vi "XY_plot_gnuplot.vi"(0 "Plot Array":cluster{dbl[], dbl[]}[](array[cluster])=[{[500.0, 500.0, 953.54, 215.0, 270.0, 320.0, 445.0, 525.0, 600.0, 675.0, 750.0, 825.0, 900.0, 960.0, 1010.0, 1060.0], [4.614524, 4.54365, 5.818368, 0.1374656, 0.6662545, 1.465458, 3.619824, 4.848976, 5.887329, 5.940571, 6.152151, 5.717487, 5.600293, 5.40069, 5.154843, 5.121789]}, {[100.0, 150.0, 215.0, 270.0, 320.0, 445.0, 525.0, 600.0, 675.0, 750.0, 825.0, 900.0, 960.0, 1010.0, 1060.0], [0.002314715, -0.00693192, 0.120417, 0.6880509, 1.519176, 3.513709, 5.065183, 6.116033, 6.096773, 5.938465, 5.593788, 5.5597, 5.387002, 5.304077, 4.887903]}] {"?" format="%.2f"; "?" format="%.2f"}, 1 "Job Directory":path=path "/G4_2_HD/Users/paulhayden/Documents/Projects/Westlakes_resolution") -> (2 "Saved Automatically?":bool, 3 "Tex Info String":string="set term epslatex\nset output \"Plot.eps\"\nset xlabel '$Distance~(m)$'\nset ylabel '$DF~(s/m^3)\\times10^6$'\nset samples 1000\nset pointsize 1.00\nset title '$B38~Centreline~Glc$' 0, 0\nset size 0.75,0.9\n\n#set key 450, -2.5833\n unset key\nset label 1 '~~~~~~~~~~~Angle~(deg)~=~0' at -100, -2.58\nset label 2 '~~~~~~~~~~~Height~(m)~=~5' at -100, -3.27\n set xrange [0 : 500] \n# set autoscale x \n set yrange [0.10000 : 7]\n# set autoscale y \n\nplot \"B38_Centreline_Glc.dat\" index 0 using 1:2 axes x1y1 title '$File=B38R~DDD.xls$' with points 1 1, \\\n\"B38_Centreline_Glc.dat\" index 1 using 1:2 axes x1y1 title '$File=B38R~DDD~1.xls$' with points 1 3", 4 "Plot data file":path)   [LabVIEW 2011]
uses:
  Gnuplot_Label.ctl
  Results_plotter_Global.vi
  <vilib>/Analysis/NI_AALBase.lvlib
  <vilib>/Analysis/NI_AALPro.lvlib
panel:
  in  "Fixed Zp":dbl format="%.2f"
  in  "Auto Zp":bool=TRUE
  in  "Put Coeff\nin Results file":bool
  in  "Case Constant\n(See Context Help)":bool
  in  "Minor Gridlines":T1(ring)
  in  "Major Gridlines":T1(ring)
  in  "Legend Position":u16(ring) items=["Auto", "top left", "top right", "bottom left", "bottom right"]
  in  "Ymax":bool=TRUE
  in  "Ymax Val":dbl
  in  "Xmax":bool=TRUE
  in  "Xmax Val":dbl
  in  "Xmin":bool=TRUE
  in  "Xmin Val":dbl
  in  "Ymin":bool=TRUE
  in  "X Log?":bool
  out "Time format?":bool
  in  "plot error bars?":bool
  out "Path":path
  in  "Show Labels?":bool
  in  "Ymin Val":dbl
  out "Final Title":string="B38 Centreline Glc"
  in  "y Log?":bool
  in  "Show Re-Run Gnuplot?":bool
  in  "Mode":T2
  in  "Wavelength?":bool
  in  "Separation":dbl=1.2
  in  "Reverse order":bool
  in  "Offset?":bool
  out "Extra range":dbl
  in  "precision":string
  out "Profile offset":dbl
  in  "Graph Height":string="0.9"
  in  "Graph width":string="0.75"
  in  "Filename Max length":i32=28
  in  "Save data analysis file":bool
  in  "Plot Title":u16(ring) items=["Title String Only", "Number of Measurements", "Date:of:Measurement", "Time:Measurement:Commenced", "Seconds:since:1st Jan", "Time::", "Raw:Data:Filename", "w1Demeaned::", "w2Demeaned::", "w3Demeaned::", "w5Demeaned::", "Ch 1:Mean:Gen (w1)", "Ch 1:Variance:Gen (w1)", "Ch 2:Mean:Gen (w2)", "Ch 2:Variance:Gen (w2)", "Ch 3:Mean:Gen (w3)", "Ch 3:Variance:Gen (w3)", "Ch 4:Mean:Gen (w5)", "Ch 4:Variance:Gen (w5)", "Tunnel3:SettlingChamber:Temperature(C)"]
  in  "Plot style":u16[](array[ring])=[0, 0, 0, 0, 0, 0, 0, 0, 0, 0, 0] items=["points", "lines", "linespoints"]
  in  "Summarise":u16(ring) items=["All Series", "w1Demeaned__", "w2Demeaned__", "w3Demeaned__", "w5Demeaned__"]
  in  "Added labels":i32[](listbox)
  out "Delta y":dbl=0.6900000000000001
  out "Y location":dbl=-2.583333333333333
  out "X location":dbl=-100.0
  in  "Plot Title":string
  in  "Show legend?":bool
  in  "Point Size":dbl=1.2 format="%.2f"
  out "No of Series":i32=2
  in  "Fit type":T3(ring)
  out "No Legend":i32=397
  out "With legend":i32=580
  in  "Save Automatically?":bool
  in  "Analysis":T4(ring)
  out "XY Graph":cluster{dbl[], dbl[]}[](graph)=[{[215.0, 270.0, 320.0, 445.0, 500.0, 500.0, 525.0, 600.0, 675.0, 750.0, 825.0, 900.0, 953.54, 960.0, 1010.0, 1060.0], [0.1374656, 0.6662545, 1.465458, 3.619824, 4.614524, 4.54365, 4.848976, 5.887329, 5.940571, 6.152151, 5.717487, 5.600293, 5.818368, 5.40069, 5.154843, 5.121789]}, {[100.0, 150.0, 215.0, 270.0, 320.0, 445.0, 525.0, 600.0, 675.0, 750.0, 825.0, 900.0, 960.0, 1010.0, 1060.0], [0.002314715, -0.00693192, 0.120417, 0.6880509, 1.519176, 3.513709, 5.065183, 6.116033, 6.096773, 5.938465, 5.593788, 5.5597, 5.387002, 5.304077, 4.887903]}]
  # "Scales"
  # "Auto"
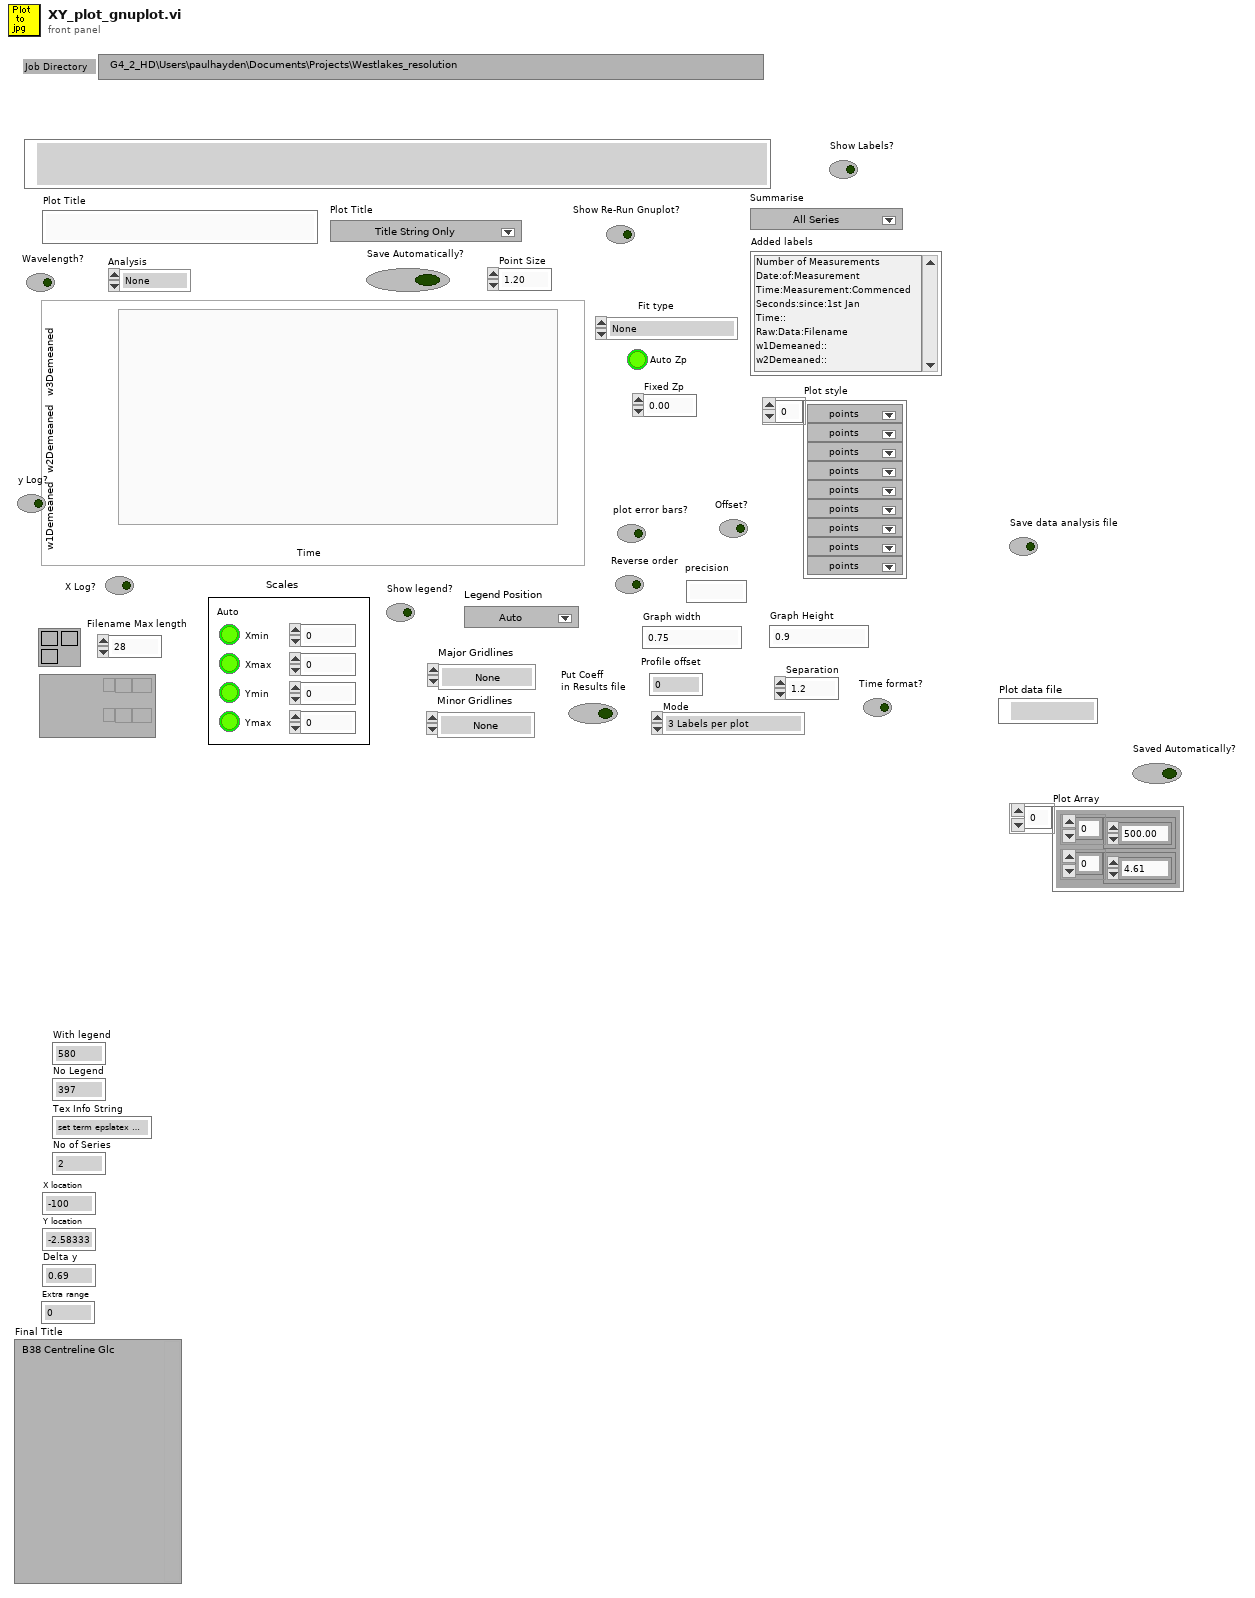
[diagram p1: front panel]
types:
  T1 = enum16{"None", "X only", "Y only", "Both X and Y"}
  T2 = typedef "Gnuplot_Label.ctl" = enum16{"3 Labels per plot", "Only Center label", "Only Bottom Label"}
  T3 = enum16{"None", "Spline", "Linear", "2nd Ploy", "3rd Poly", "4th Poly", "Gauss Lat", "Gauss vert", "Gauss Vert with 2 sig", "Guass glc"}
  T4 = enum16{"None", "% change", "Spectrum", "Norm Spec"}
  T5 = enum16{"None", "Lines", "Linespoints", "Spline", "Linear", "2nd Ploy", "3rd Poly", "4th Poly", "Gauss Lat", "Gauss vert", "Guass glc"}
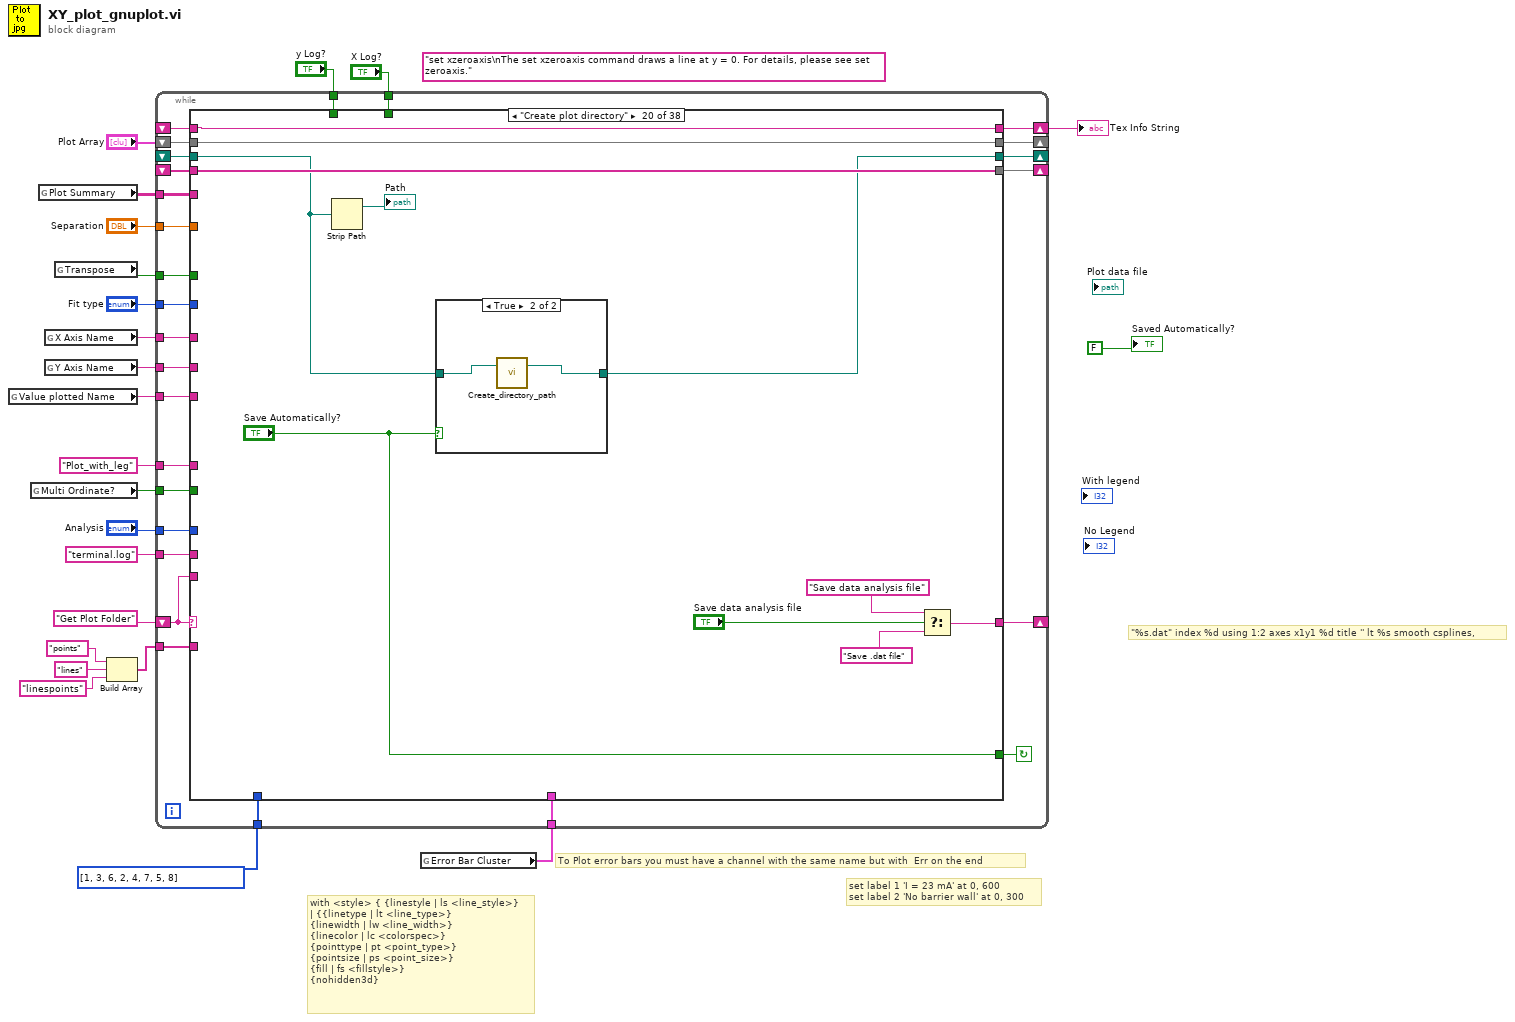
[diagram p0: block diagram]
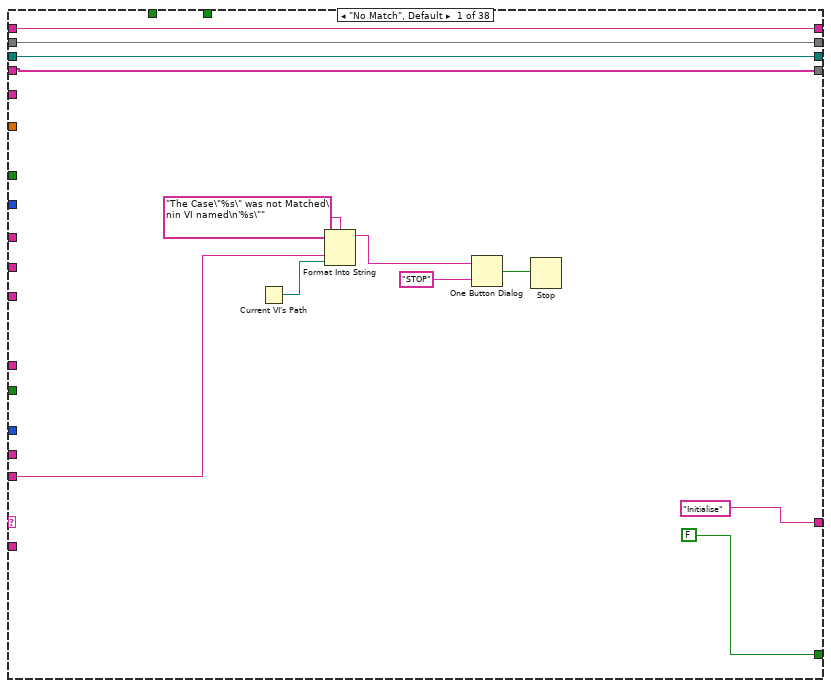
[diagram p2: hidden frame]
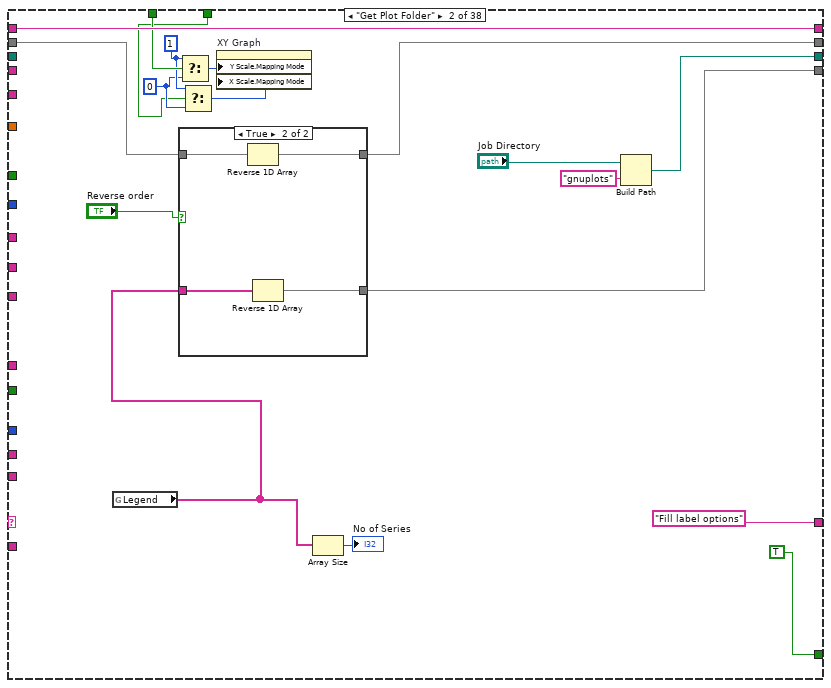
[diagram p3: hidden frame]
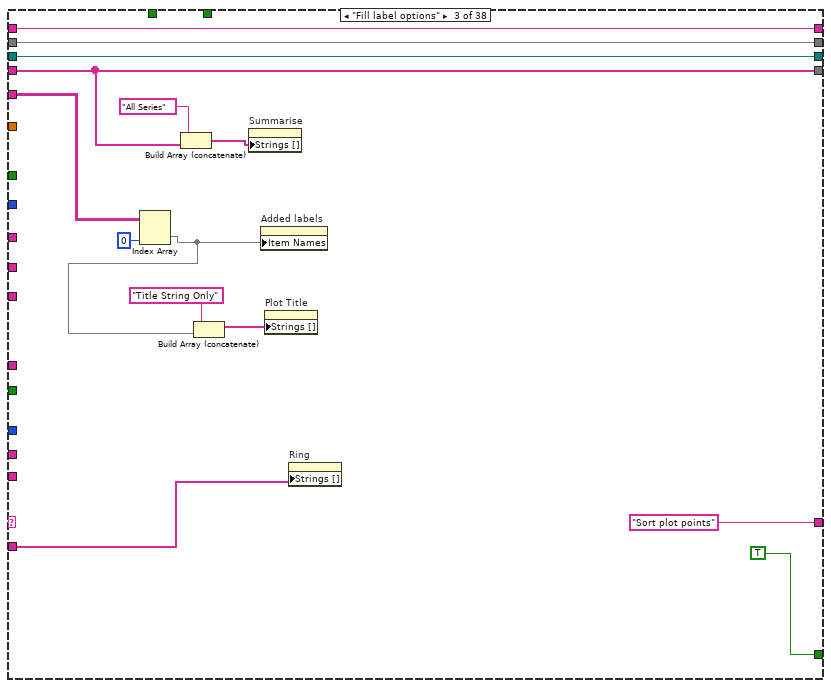
[diagram p5: hidden frame]
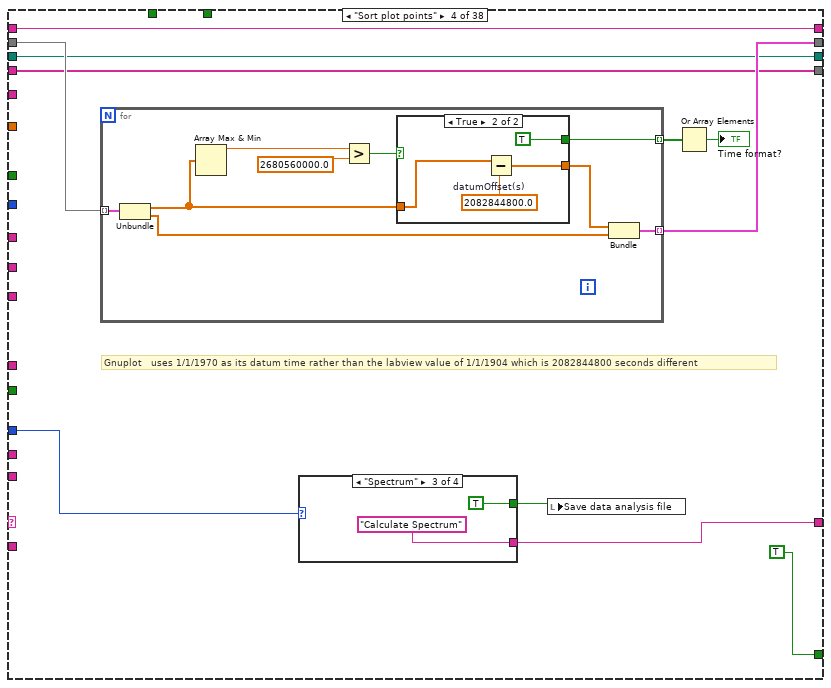
[diagram p6: hidden frame]
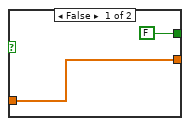
[diagram p7: hidden frame]
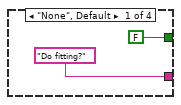
[diagram p8: hidden frame]
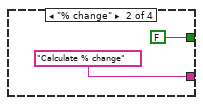
[diagram p9: hidden frame]
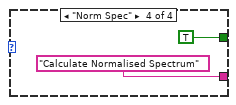
[diagram p10: hidden frame]
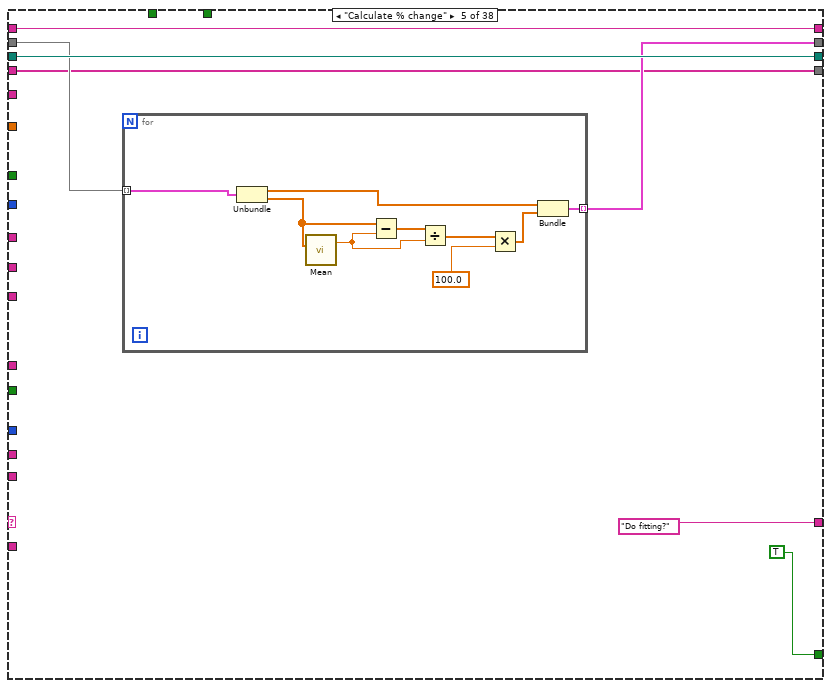
[diagram p11: hidden frame]
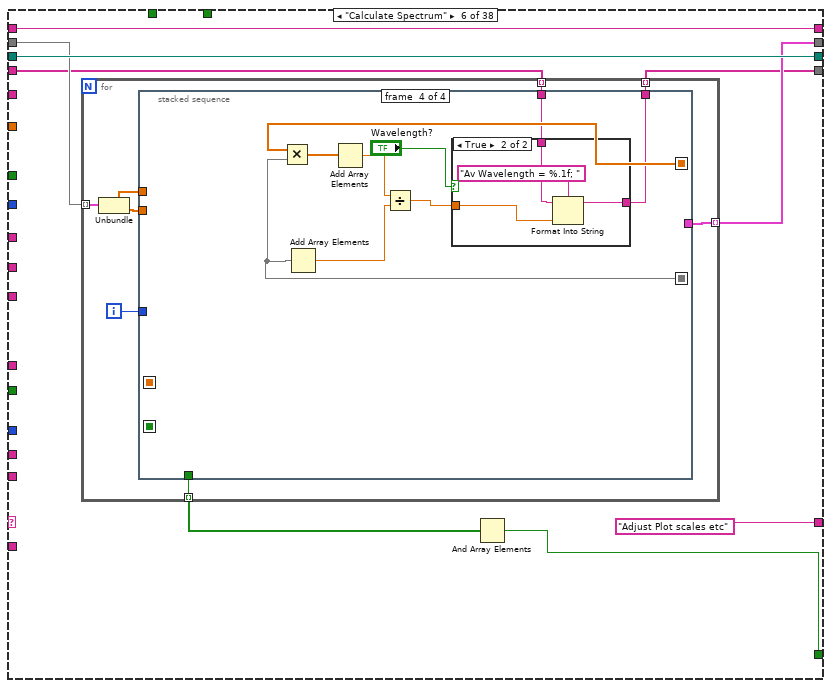
[diagram p12: hidden frame]
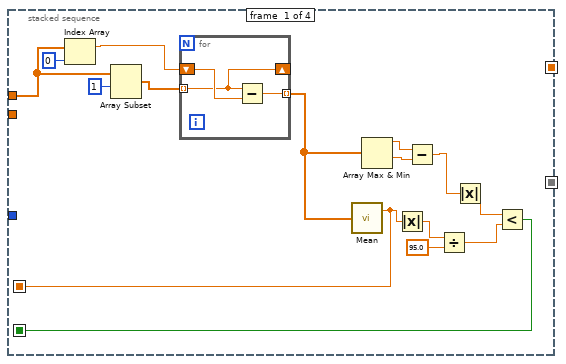
[diagram p13: hidden frame]
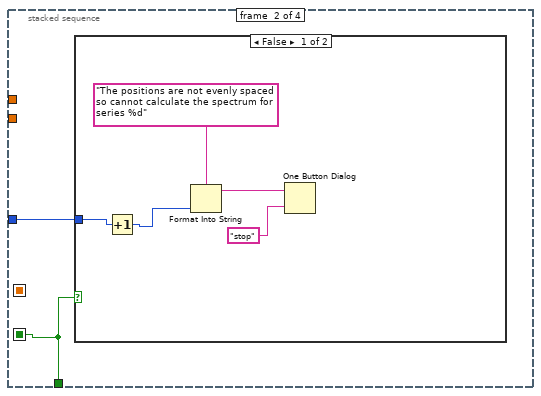
[diagram p14: hidden frame]
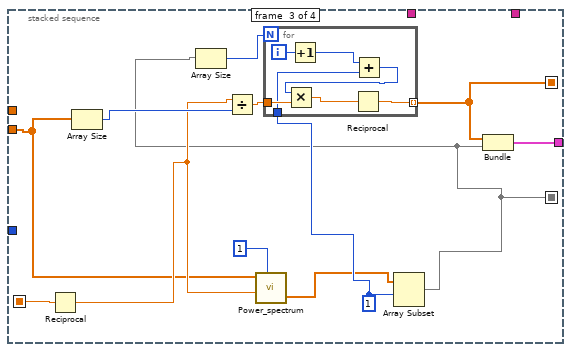
[diagram p16: hidden frame]
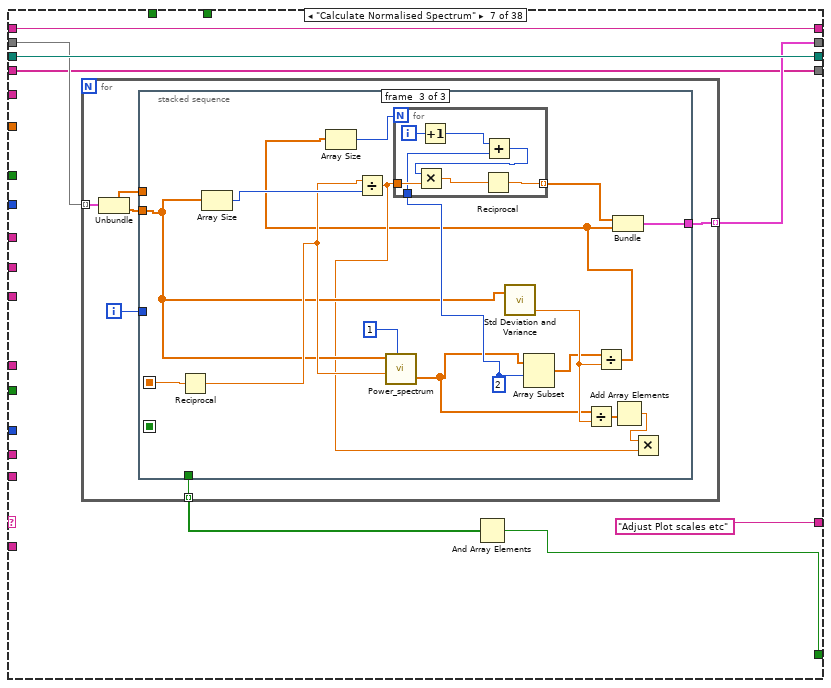
[diagram p18: hidden frame]
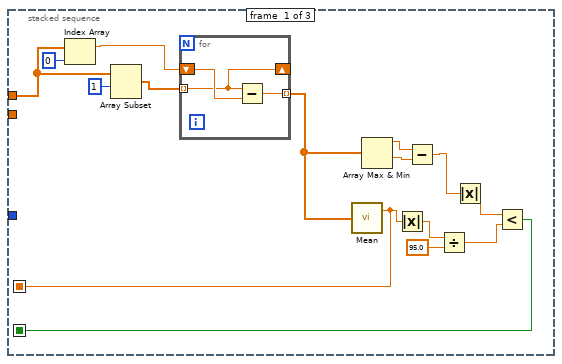
[diagram p19: hidden frame]
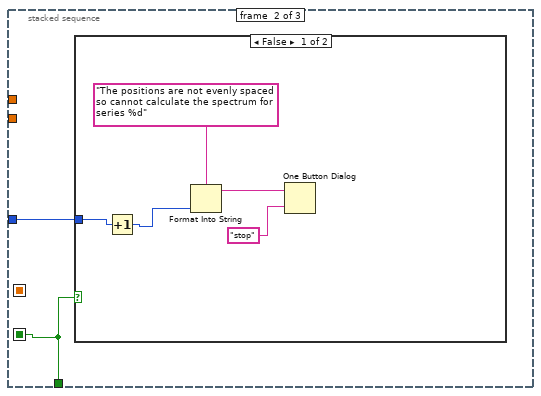
[diagram p20: hidden frame]
diagram:
  (unwired) "set xzeroaxis\nThe set xzeroaxis command draws a line at y = 0. For details, please see set zeroaxis."
  # "\"%s.dat\" index %d using 1:2 axes x1y1 %d title '' lt %s smooth csplines,"
  # "with <style> { {linestyle | ls <line_style>} \n| {{linetype | lt <line_type>} \n{linewidth | lw <line_width>} \n{linecolor | lc <colorspec>} \n{pointtype | pt <point_type>} \n{pointsize | ps <point_size>} \n{fill | fs <fillstyle>} \n{nohidden3d}"
  # "To Plot error bars you must have a channel with the same name but with  Err on the end"
  # "set label 1 'I = 23 mA' at 0, 600\nset label 2 'No barrier wall' at 0, 300"
  n1 = global read "Results_plotter_Global.vi" "Value plotted Name"() -> (w19:string)
  n2 = global read "Results_plotter_Global.vi" "Multi Ordinate?"() -> (w1:bool)
  n3 = global read "Results_plotter_Global.vi" "Plot Summary"() -> (w22:string[][])
  n4 = global read "Results_plotter_Global.vi" "X Axis Name"() -> (w21:string)
  n5 = global read "Results_plotter_Global.vi" "Y Axis Name"() -> (w20:string)
  n6 = global read "Results_plotter_Global.vi" "Transpose"() -> (w2:bool)
  n7 = Build Array("points", "lines", "linespoints") -> (w9:string[])
  n8 = global read "Results_plotter_Global.vi" "Error Bar Cluster"() -> (w4:cluster{string[]}[])
  n9 = while {
    shift-left: "Get Plot Folder" -> [w48]
    shift-right: [w49] -> _
    tunnel: w22 -> [w47]
    shift-right: [w46] -> _
    shift-left: _ -> [w45]
    tunnel: "Analysis" -> [w44]
    tunnel: w21 -> [w43]
    tunnel: w20 -> [w42]
    tunnel: w19 -> [w41]
    shift-right: [w39] -> _
    shift-left: "Plot Array" -> [w40]
    shift-right: [w37] -> w17
    shift-left: _ -> [w38]
    tunnel: "Plot_with_leg" ("name or relative path") -> [w36]
    tunnel: "Fit type" -> [w35]
    shift-right: [w34] -> _
    shift-left: _ -> [w33]
    tunnel: "terminal.log" -> [w32]
    tunnel: w9 -> [w31]
    tunnel: i32[] [1, 3, 6, 2, 4, 7, 5, 8] ("Plot style") -> [w30]
    tunnel: "Separation" -> [w29]
    tunnel: "y Log?" -> [w28]
    tunnel: w4 -> [w27]
    tunnel: "X Log?" -> [w26]
    tunnel: w2 -> [w25]
    tunnel: w1 -> [w24]
    stop <- w50 continue-if-true
    n10 = case shown="\"Create plot directory\"" w48 {
      tunnel: [FALSE TRUE TRUE ("Top Level") TRUE TRUE w153 w226 TRUE TRUE TRUE ("Top Level") TRUE ("Top Level") TRUE ("Top Level") TRUE ("Top Level") TRUE ("Top Level") TRUE ("Top Level") TRUE ("Top Level") TRUE ("Top Level") TRUE ("Top Level") TRUE ("Top Level") "Save Automatically?" w743 w816 TRUE ("Top Level") TRUE ("Top Level") TRUE ("Top Level") TRUE ("Top Level") TRUE ("Top Level") TRUE ("Top Level") TRUE ("Top Level") TRUE ("Top Level") TRUE ("Top Level") TRUE ("Top Level") TRUE ("Top Level") TRUE ("Top Level") TRUE ("Top Level") w1674 FALSE ("Top Level") FALSE ("Top Level")] -> w50
      tunnel: ["Initialise" "Fill label options" "Sort plot points" w104 "Do fitting?" "Adjust Plot scales etc" "Adjust Plot scales etc" "Adjust Plot scales etc" "Add fitted line styles" "Adjust Plot scales etc" w383 "Fill Second legend" "Fill Second legend" "Fill Second legend" "Calculate plot max and min values" "Sort out plot title" w579 w681 "Create plot directory" w726 w742 w815 w952 "Edit Legend names" w1151 "Labels?" ("t") "Labels?" ("t") w1323 w1348 "Plot Command" "Write gnuplot file" ("t") "Execute shell script" ("t") "Has pdf been generated?" ("t") w1651 "Input Fit Coefficients into results file?" "Read Fit Coefficients" ("t") "End" ("t") "End" ("t")] -> w49
      tunnel: w48 -> [w57 _ _ _ _ _ _ _ _ _ _ _ _ _ _ _ _ _ _ _ _ _ _ _ _ _ _ _ _ _ _ _ _ _ _ _ _ _]
      tunnel: w47 -> [_ _ w100 _ _ _ _ _ _ _ _ _ _ _ _ _ w589 _ _ _ w741 w814 _ _ _ _ _ _ w1347 _ _ _ _ _ _ _ _ _]
      tunnel: [w54 w77 w94 w108 w139 w158 w232 w293 w308 w369 w396 w430 w439 w451 w478 w512 w581 w682 w692 w728 w744 w817 w979 w1019 w1166 w1228 w1291 w1330 w1354 w1477 w1509 w1636 w1644 w1657 w1668 w1679 w1697 w1772] -> w46
      tunnel: w45 -> [w54 _ w94 w108 w139 w158 w232 w293 w308 w369 w396 w430 w439 w451 w474 w512 w580 w678 w699 w723 w744 w817 w979 w1019 w1166 w1228 w1291 w1330 w1354 w1477 w1509 w1636 w1644 w1657 w1668 w1679 w1697 w1772]
      tunnel: w44 -> [_ _ _ w105 _ _ _ _ _ _ w384 _ _ w445 _ _ _ w669 _ _ w737 w809 w976 _ _ _ _ _ _ _ _ _ _ _ _ _ _ _]
      tunnel: w43 -> [_ _ _ _ _ _ _ _ w299 _ _ w426 w438 _ _ _ _ _ _ _ w740 w813 w974 _ _ _ _ _ _ _ _ _ _ _ _ _ _ _]
      tunnel: w42 -> [_ _ _ _ _ _ _ _ w298 _ _ w425 w437 w450 _ _ _ _ _ _ w739 w812 w975 _ _ _ _ _ _ _ _ _ _ _ _ _ _ _]
      tunnel: w41 -> [_ _ _ _ _ _ _ _ _ _ _ _ _ _ _ _ _ _ _ _ w736 _ _ _ _ _ _ _ _ _ _ _ _ _ _ _ w1691 _]
      tunnel: w40 -> [w53 w72 w95 w110 w138 w157 w231 w289 w304 w368 w382 w429 w436 w449 w477 w509 w596 w680 w702 w731 w735 w811 w980 w1006 w1161 w1220 w1284 w1327 w1349 w1478 w1511 w1642 w1649 w1664 w1673 w1683 w1686 w1777]
      tunnel: [w53 w71 w95 w109 w137 w156 w230 w289 w297 w368 w382 w429 w436 w449 w477 w509 w596 w680 w702 w731 w735 w808 w980 w1006 w1161 w1220 w1284 w1327 w1349 w1478 w1511 w1642 w1649 w1664 w1673 w1683 w1686 w1777] -> w39
      tunnel: w38 -> [w52 w76 w96 w107 w136 w155 w229 w292 w307 w366 w385 w428 w435 w448 w476 w513 w591 w679 w701 w730 w745 w818 _ w1017 w1165 w1224 w1287 w1318 w1351 w1473 w1507 w1631 w1647 w1662 w1671 w1681 w1700 w1775]
      tunnel: [w52 w76 w96 w107 w136 w155 w229 w292 w307 w366 w385 w428 w435 w448 w476 w513 w591 w679 w701 w730 w745 w818 w955 w1015 w1165 w1225 w1288 w1317 w1352 w1469 w1506 w1631 w1647 w1662 w1671 w1681 w1700 w1775] -> w37
      tunnel: w36 -> [_ _ _ _ _ _ _ _ _ _ _ _ _ _ _ _ _ _ _ _ _ _ _ _ _ _ _ _ _ _ _ _ _ _ _ _ _ _]
      tunnel: w35 -> [_ _ _ _ _ _ _ w290 w306 _ w387 _ _ _ _ _ _ _ _ _ _ _ w953 w1021 _ _ _ _ _ w1442 w1498 _ _ _ _ w1678 w1693 _]
      tunnel: [w51 w70 w92 w106 w135 w151 w228 w291 w301 w365 w389 w427 w434 w447 w475 w511 w595 w677 w700 w729 w738 w810 w978 w1022 w1167 w1227 w1290 w1329 w1353 w1463 w1508 w1637 w1648 w1663 w1672 w1682 w1701 w1776] -> w34
      tunnel: w33 -> [w51 _ w92 w106 w135 w152 w228 w291 w302 w365 w389 w427 w434 w447 w475 w511 w595 w677 w700 w729 w738 w810 w978 w1022 w1168 w1227 w1290 w1329 w1353 w1463 w1508 w1637 w1648 w1663 w1672 w1682 w1701 w1776]
      tunnel: w32 -> [_ _ _ _ _ _ _ _ _ _ _ _ _ _ _ _ _ _ _ _ _ _ _ _ _ _ _ _ _ _ _ _ w1643 _ _ _ _ w1770]
      tunnel: w31 -> [_ _ w90 _ _ _ _ _ _ _ _ _ _ _ _ _ _ _ _ _ _ _ _ _ _ _ _ _ _ _ _ _ _ _ _ _ _ _]
      tunnel: w30 -> [_ _ _ _ _ _ _ _ _ _ _ _ _ _ _ _ _ _ _ _ _ _ _ _ _ _ _ _ _ _ w1496 w1633 _ _ _ _ _ _]
      tunnel: w29 -> [_ _ _ _ _ _ _ _ _ _ _ _ _ _ _ _ _ _ _ _ _ w807 _ _ w1160 _ _ _ _ w1460 _ _ _ _ _ _ _ _]
      tunnel: w28 -> [_ w69 _ _ _ _ _ _ _ _ _ _ _ _ _ _ _ _ _ _ _ _ _ _ _ w1199 w1271 _ w1346 w1457 _ _ _ _ _ _ _ _]
      tunnel: w27 -> [_ _ _ _ _ _ _ _ _ _ _ _ _ _ _ w482 _ _ _ _ _ w806 _ _ _ _ _ _ _ _ w1495 _ _ _ _ _ _ _]
      tunnel: w26 -> [_ w64 _ _ _ _ _ _ _ _ _ _ _ _ _ _ _ _ _ _ _ _ _ _ _ w1192 _ _ w1345 w1452 _ _ _ _ _ _ _ _]
      tunnel: w25 -> [_ _ _ _ _ _ _ _ _ _ _ _ _ _ _ w480 _ _ _ _ _ w805 _ w1007 _ _ _ _ _ w1447 w1491 _ _ _ _ _ _ _]
      tunnel: w24 -> [_ _ _ _ _ _ _ _ _ _ _ _ _ _ _ _ _ _ _ _ _ _ _ _ _ _ _ _ _ _ _ _ _ _ _ _ _ _]
      frame "No Match", Default {
        n11 = Current VI's Path() -> (path=w56:path)
        n12 = Format Into String(format string="The Case\"%s\" was not Matched\nin VI named\n'%s\"" ("Format String"), w57, w56) -> (resulting string=w60:string)  [unwired: 2 in, 1 out]
        n13 = One Button Dialog(message=w60, button name ("OK")="STOP") -> (true=w58:bool)
        n14 = Stop(stop? (T)=w58) -> ()
      }
      frame "Get Plot Folder" {
        w65 = u8 0 ("f")
        w66 = u8 1 ("Y Scale.Mapping Mode")
        n15 = global read "Results_plotter_Global.vi" "Legend"() -> (w63:string[])
        n16 = case shown="True" "Reverse order" {
          tunnel: w72 -> [w82 w86]
          tunnel: [w82 w85] -> w71
          tunnel: w63 -> [w81 w84]
          tunnel: [w81 w83] -> w70
          frame False {
          }
          frame True {
            n17 = Reverse 1D Array(array=w86) -> (reversed array=w85:cluster{"Output":dbl[], dbl[]}[])
            n18 = Reverse 1D Array(array=w84) -> (reversed array=w83:string[])
          }
        }
        n19 = Select(t=w66, s=w69, f=w65) -> (s? t:f=w68:u8)
        n20 = Select(t=w66, s=w64, f=w65) -> (s? t:f=w67:u8)
        n21 = property on="XY Graph" class="XYGraph (strict)"("Y Scale.Mapping Mode"=w68, "X Scale.Mapping Mode"=w67) -> ()  [unwired: 2 in, 2 out]
        n22 = Array Size(array=w63) -> (size(s)=→"No of Series":i32)
        n23 = Build Path(base path="Job Directory", name or relative path="gnuplots") -> (appended path=w77:path)
      }
      frame "Fill label options" {
        n24 = Index Array(array=w100, index (col)=0 ("disabled index (col)")) -> (element=w88:string[])  [unwired: 1 in]
        n25 = Build Array (concatenate)("All Series", w92) -> (w93:string[])
        n26 = Build Array (concatenate)("Title String Only", w88) -> (w87:string[])
        n27 = property on="Summarise" class="Ring (strict)"("Strings []"=w93) -> ()  [unwired: 2 in, 2 out]
        n28 = property on="Added labels" class="LstBox (strict)"("Item Names"=w88) -> ()  [unwired: 2 in, 2 out]
        n29 = property on="Plot Title" class="Ring (strict)"("Strings []"=w87) -> ()  [unwired: 2 in, 2 out]
        n30 = property on="Ring" class="Ring (strict)"("Strings []"=w90) -> ()  [unwired: 2 in, 2 out]
      }
      frame "Sort plot points" {
        # "Gnuplot   uses 1/1/1970 as its datum time rather than the labview value of 1/1/1904 which is 2082844800 seconds different"
        n31 = for {
          tunnel: w110 -> [w119] mode=indexing
          tunnel: [w120] -> w109 mode=indexing
          tunnel: [w112] -> w102 mode=indexing
          n32 = Unbundle(w119) -> ("Output"=w115:dbl[], w116:dbl[])
          n33 = Array Max & Min(array=w115) -> (max value=w118:dbl)  [unwired: 3 out]
          n34 = Greater?(x=w118, y=2680560000.0) -> (0:w113:bool)
          n35 = case shown="True" w113 {
            tunnel: w115 -> [w122 w126]
            tunnel: [w122 w124] -> w114
            tunnel: [FALSE TRUE] -> w112
            frame False {
            }
            frame True {
              w125 = 2082844800.0  # datumOffset(s)
              n36 = Subtract(x=w126, y=w125) -> (x-y=w124:dbl[])
            }
          }
          n37 = Bundle("Output"=w114, w116) -> (w120:cluster{"Output":dbl[], dbl[]})  [unwired: 1 out]
        }
        n38 = case shown="\"Spectrum\"" w105 {
          tunnel: ["Do fitting?" "Calculate % change" "Calculate Spectrum" "Calculate Normalised Spectrum"] -> w104
          tunnel: [FALSE ("Save data analysis file") FALSE ("Save data analysis file") TRUE ("Save data analysis file") TRUE ("Save data analysis file")] -> w103
          frame "None", Default {
          }
          frame "% change" {
          }
          frame "Spectrum" {
          }
          frame "Norm Spec" {
          }
        }
        n39 = local write "Save data analysis file"(w103) -> ()
        n40 = Or Array Elements(Boolean array=w102) -> (logical OR=→"Time format?":bool)
      }
      frame "Calculate % change" {
        n41 = for {
          tunnel: w138 -> [w150] mode=indexing
          tunnel: [w142] -> w137 mode=indexing
          n42 = Unbundle(w150) -> ("Output"=w144:dbl[], w149:dbl[])
          n43 = call <vilib>:"Mean.vi"("X"=w149) -> ("mean"=w147:dbl)  [unwired: 1 out]
          n44 = Subtract(x=w149, y=w147) -> (x-y=w148:dbl[])
          n45 = Divide(x=w148, y=w147) -> (x/y=w146:dbl[])
          n46 = Multiply(x=w146, y=100.0) -> (x*y=w143:dbl[])
          n47 = Bundle("Output"=w144, w143) -> (w142:cluster{"Output":dbl[], dbl[]})  [unwired: 1 out]
        }
      }
      frame "Calculate Spectrum" {
        n48 = for {
          tunnel: w157 -> [w166] mode=indexing
          tunnel: [w167] -> w156 mode=indexing
          tunnel: [w162] -> w154 mode=indexing
          tunnel: w152 -> [w161] mode=indexing
          tunnel: [w160] -> w151 mode=indexing
          i -> [w163]
          n49 = Unbundle(w166) -> ("Output"=w164:dbl[], w165:dbl[])
          n50 = stacked-sequence {
            seq-local: [w169 _ _ _] -> [_ _ w199 _]
            seq-local: [w168 _ _ _] -> [_ w186 _ _]
            seq-local: [_ _ w194 _] -> [_ _ _ w219]
            seq-local: [_ _ w193 _] -> [_ _ _ w220]
            tunnel: [_ _ w204 _] -> w167
            tunnel: w165 -> [_ _ w197 _]
            tunnel: w164 -> [w180 _ _ _]
            tunnel: w163 -> [_ w187 _ _]
            tunnel: [_ w186 _ _] -> w162
            tunnel: w161 -> [_ _ _ w215]
            tunnel: [_ _ _ w213] -> w160
            frame #0 {
              n51 = Index Array(array=w180, index=0) -> (element=w179:dbl)
              n52 = Array Subset(array=w180, index=1) -> (w178:dbl[])  [unwired: 1 in]
              n53 = for {
                shift-right: [w184] -> _
                shift-left: w179 -> [w185]
                tunnel: w178 -> [w184] mode=indexing
                tunnel: [w183] -> w175 mode=indexing
                n54 = Subtract(x=w184, y=w185) -> (x-y=w183:dbl)
              }
              n55 = call <vilib>:"Mean.vi"("X"=w175) -> ("mean"=w169:dbl)  [unwired: 1 out]
              n56 = Array Max & Min(array=w175) -> (max value=w177:dbl, min value=w176:dbl)  [unwired: 2 out]
              n57 = Absolute Value(x=w169) -> (abs(x)=w172:dbl)
              n58 = Subtract(x=w177, y=w176) -> (x-y=w174:dbl)
              n59 = Divide(x=w172, y=95.0) -> (x/y=w170:dbl)
              n60 = Absolute Value(x=w174) -> (abs(x)=w173:dbl)
              n61 = Less?(x=w173, y=w170) -> (x < y?=w168:bool)
            }
            frame #1 {
              n62 = case shown="False" w186 {
                tunnel: w187 -> [w192 _]
                frame False {
                  n63 = Increment(x=w192) -> (x+1=w191:i32)
                  n64 = Format Into String(format string="The positions are not evenly spaced so cannot calculate the spectrum for series %d", w191) -> (resulting string=w189:string)  [unwired: 2 in, 1 out]
                  n65 = One Button Dialog(message=w189, button name ("OK")="stop") -> ()  [unwired: 1 out]
                }
                frame True {
                }
              }
            }
            frame #2 {
              w200 = 1 ("index")
              n66 = Reciprocal(x=w199) -> (1/x=w198:dbl)
              n67 = Array Size(array=w197) -> (size(s)=w201:i32)
              n68 = Divide(x=w198, y=w201) -> (x/y=w195:dbl)
              n69 = call "Power_spectrum.vi"("U"=w197, "Sampling frequency"=w198, "Block No"=1) -> ("Spectrum output array"=w196:dbl[])  [unwired: 1 in, 2 out]
              n70 = Array Subset(array=w196, index=w200) -> (w193:dbl[])  [unwired: 1 in]
              n71 = Array Size(array=w193) -> (size(s)=w203:i32)
              n72 = for {
                N: w203 -> [_]
                tunnel: [w208] -> w194 mode=indexing
                tunnel: w195 -> [w210]
                tunnel: w200 -> [w206]
                i -> [w211]
                n73 = Increment(x=w211) -> (x+1=w207:i32)
                n74 = Add(x=w207, y=w206) -> (x+y=w205:i32)
                n75 = Multiply(x=w205, y=w210) -> (x*y=w209:dbl)
                n76 = Reciprocal(x=w209) -> (1/x=w208:dbl)
              }
              n77 = Bundle(w194, w193) -> (w204:cluster{dbl[], dbl[]})  [unwired: 1 out]
            }
            frame #3 {
              n78 = Multiply(x=w219, y=w220) -> (x*y=w218:dbl[])
              n79 = Add Array Elements(numeric array=w220) -> (sum=w216:dbl)
              n80 = Add Array Elements(numeric array=w218) -> (sum=w217:dbl)
              n81 = Divide(x=w217, y=w216) -> (x/y=w214:dbl)
              n82 = case shown="True" "Wavelength?" {
                tunnel: w215 -> [w221 w225]
                tunnel: w214 -> [_ w224]
                tunnel: [w221 w222] -> w213
                frame False {
                }
                frame True {
                  n83 = Format Into String(format string="Av Wavelength = %.1f; ", initial string=w225, w224) -> (resulting string=w222:string)  [unwired: 1 in, 1 out]
                }
              }
            }
          }
        }
        n84 = And Array Elements(Boolean array=w154) -> (logical AND=w153:bool)
      }
      frame "Calculate Normalised Spectrum" {
        n85 = for {
          tunnel: w231 -> [w238] mode=indexing
          tunnel: [w239] -> w230 mode=indexing
          tunnel: [w234] -> w227 mode=indexing
          i -> [w235]
          n86 = Unbundle(w238) -> ("Output"=w236:dbl[], w237:dbl[])
          n87 = stacked-sequence {
            seq-local: [w241 _ _] -> [_ _ w274]
            seq-local: [w240 _ _] -> [_ w258 _]
            tunnel: [_ _ w280] -> w239
            tunnel: w237 -> [_ _ w272]
            tunnel: w236 -> [w252 _ _]
            tunnel: w235 -> [_ w259 _]
            tunnel: [_ w258 _] -> w234
            frame #0 {
              n88 = Index Array(array=w252, index=0) -> (element=w251:dbl)
              n89 = Array Subset(array=w252, index=1) -> (w250:dbl[])  [unwired: 1 in]
              n90 = for {
                shift-right: [w256] -> _
                shift-left: w251 -> [w257]
                tunnel: w250 -> [w256] mode=indexing
                tunnel: [w255] -> w247 mode=indexing
                n91 = Subtract(x=w256, y=w257) -> (x-y=w255:dbl)
              }
              n92 = call <vilib>:"Mean.vi"("X"=w247) -> ("mean"=w241:dbl)  [unwired: 1 out]
              n93 = Array Max & Min(array=w247) -> (max value=w249:dbl, min value=w248:dbl)  [unwired: 2 out]
              n94 = Absolute Value(x=w241) -> (abs(x)=w244:dbl)
              n95 = Subtract(x=w249, y=w248) -> (x-y=w246:dbl)
              n96 = Divide(x=w244, y=95.0) -> (x/y=w242:dbl)
              n97 = Absolute Value(x=w246) -> (abs(x)=w245:dbl)
              n98 = Less?(x=w245, y=w242) -> (x < y?=w240:bool)
            }
            frame #1 {
              n99 = case shown="False" w258 {
                tunnel: w259 -> [w264 _]
                frame False {
                  n100 = Increment(x=w264) -> (x+1=w263:i32)
                  n101 = Format Into String(format string="The positions are not evenly spaced so cannot calculate the spectrum for series %d", w263) -> (resulting string=w261:string)  [unwired: 2 in, 1 out]
                  n102 = One Button Dialog(message=w261, button name ("OK")="stop") -> ()  [unwired: 1 out]
                }
                frame True {
                }
              }
            }
            frame #2 {
              w275 = 2 ("index")
              n103 = Reciprocal(x=w274) -> (1/x=w273:dbl)
              n104 = Array Size(array=w272) -> (size(s)=w276:i32)
              n105 = Divide(x=w273, y=w276) -> (x/y=w267:dbl)
              n106 = call "Power_spectrum.vi"("U"=w272, "Sampling frequency"=w273, "Block No"=1) -> ("Spectrum output array"=w270:dbl[])  [unwired: 1 in, 2 out]
              n107 = call <vilib>:"Std Deviation and Variance.vi"("X"=w272) -> ("variance"=w271:dbl)  [unwired: 1 in, 2 out]
              n108 = Array Subset(array=w270, index=w275) -> (w266:dbl[])  [unwired: 1 in]
              n109 = Divide(x=w270, y=w271) -> (x/y=w269:dbl[])
              n110 = Divide(x=w266, y=w271) -> (x/y=w265:dbl[])
              n111 = Array Size(array=w265) -> (size(s)=w279:i32)
              n112 = for {
                N: w279 -> [_]
                tunnel: [w284] -> w278 mode=indexing
                tunnel: w267 -> [w286]
                tunnel: w275 -> [w282]
                i -> [w287]
                n113 = Increment(x=w287) -> (x+1=w283:i32)
                n114 = Add(x=w283, y=w282) -> (x+y=w281:i32)
                n115 = Multiply(x=w281, y=w286) -> (x*y=w285:dbl)
                n116 = Reciprocal(x=w285) -> (1/x=w284:dbl)
              }
              n117 = Bundle(w278, w265) -> (w280:cluster{dbl[], dbl[]})  [unwired: 1 out]
              n118 = Add Array Elements(numeric array=w269) -> (sum=w268:dbl)
              n119 = Multiply(x=w268, y=w267) -> ()  [unwired: 1 out]
            }
          }
        }
        n120 = And Array Elements(Boolean array=w227) -> (logical AND=w226:bool)
      }
      frame "Do fitting?" {
        n121 = case shown="\"None\"" w290 {
          tunnel: ["Adjust Plot scales etc" "Poly fit to data"] -> _
          frame "None" {
          }
          frame "Linear", Default {
          }
        }
      }
      frame "Poly fit to data" {
        n122 = case shown="\"None\", Default" w306 {
          tunnel: [0 ("polynomial order") 1 ("polynomial order") 2 ("polynomial order") 3 ("polynomial order") 4 ("polynomial order")] -> w305
          frame "None", Default {
          }
          frame "Linear" {
          }
          frame "2nd Ploy" {
          }
          frame "3rd Poly" {
          }
          frame "4th Poly" {
          }
        }
        n123 = for {
          tunnel: w304 -> [w328] mode=indexing
          tunnel: [w329] -> w303 mode=indexing
          tunnel: w305 -> [w327]
          tunnel: [w322] -> w300 mode=indexing
          tunnel: w299 -> [w321]
          tunnel: w298 -> [w320]
          w326 = 8  # Enhancement factor
          n124 = Unbundle(w328) -> ("Output"=w319:dbl[], w318:dbl[])
          n125 = call <vilib>:"General Polynomial Fit.vi"("Y"=w318, "polynomial order"=w327, "X"=w319) -> ("Polynomial Coefficients"=w316:dbl[])  [unwired: 9 in, 3 out]
          n126 = case shown="False" "Case Constant\n(See Context Help)" {
            tunnel: [w332 w347] -> w323
            tunnel: [w343 w348] -> w322
            tunnel: w321 -> [w345 _]
            tunnel: w320 -> [w344 _]
            tunnel: w319 -> [w340 _]
            tunnel: w318 -> [w337 _]
            tunnel: w316 -> [_ w347]
            frame False {
              w339 = 0.99 ("Voltage")
              n127 = Build Array (concatenate)(w339, w340) -> (w342:dbl[])
              n128 = Build Array (concatenate)(nan ("Voltage"), w337) -> (w341:dbl[])
              n129 = call "Curve_Fit_ph.vi"("Values In"=w341, "No of points to fit (3)"=4, "Positions"=w342) -> ("Values Out"=w336:dbl[], "Polynomial Fit Coefficients"=w332:dbl[])  [unwired: 1 in]
              n130 = Index Array(array=w336, index=0) -> (element=w334:dbl)
              n131 = call "Number_2_string.vi"("precision"="2", "number"=w334) -> ("String"=w330:string)
              n132 = Format Into String(format string="When %s=%.2f ; %s=%s", w345, w339, w344, w330) -> (resulting string=w343:string)  [unwired: 2 in, 1 out]
            }
            frame True {
              n133 = for {
                shift-right: [w350] -> w348
                shift-left: "" -> [w351]
                tunnel: w347 -> [w354] mode=indexing
                i -> [w355]
                n134 = call "Number_2_string.vi"("number"=w354) -> ("String"=w352:string)  [unwired: 1 in]
                n135 = case shown="0, Default" w355 {
                  tunnel: [w356] -> w353
                  tunnel: w352 -> [w358]
                  frame 0, Default {
                    n136 = Concatenate Strings(w358, " ") -> (w356:string)
                  }
                }
                n137 = Concatenate Strings(w351, w353) -> (w350:string)
              }
            }
          }
          n138 = call "Enhance_No_of_points.vi"("Enhancement factor"=w326, "Input"=w319) -> ("Output"=w325:dbl[])  [unwired: 3 out]
          n139 = for {
            tunnel: w323 -> [w361]
            tunnel: w325 -> [w360] mode=indexing
            tunnel: [w359] -> w324 mode=indexing
            n140 = call "Polynomial_convert.vi"("Calib constants"=w361, "Voltage"=w360) -> ("Eng Values"=w359:dbl)  [unwired: 4 out]
          }
          n141 = Bundle("Output"=w325, w324) -> (w329:cluster{"Output":dbl[], dbl[]})  [unwired: 1 out]
        }
        n142 = Build Array (concatenate)(w302, w300) -> (w301:string[])
        n143 = Build Array (concatenate)(w304, w303) -> (w297:cluster{"Output":dbl[], dbl[]}[])
        n144 = local write "XY Graph"(w297) -> ()
      }
      frame "Add fitted line styles" {
        n145 = local read "No of Series"() -> (w362:i32)
        n146 = Array Subset(array=w365, index=w362) -> (w364:string[])  [unwired: 1 in]
        n147 = for {
          tunnel: w364 -> [w373] mode=indexing
          tunnel: u8 2 ("Plot.Plot Interpolation") -> [w379]
          tunnel: w362 -> [w375]
          i -> [w376]
          w381 = u32 0
          n148 = Concatenate Strings(w373, "  " ("string")) -> (w371:string)
          n149 = Add(x=w375, y=w376) -> (x+y=w374:i32)
          n150 = Quotient & Remainder(x=w376, y=4) -> (x-y*floor(x/y)=w377:i32)  [unwired: 1 out]
          n151 = property on="XY Graph" class="XYGraph (strict)"("Active Plot"=w374, "Plot.Plot Name"=w371, "Plot.Fill/Point Color"=w381, "Plot.Plot Color"=w381, "Plot.Point Style"=u8 0, "Plot.Line Style"=w377, "Plot.Plot Interpolation"=w379) -> ()  [unwired: 2 in, 2 out]
        }
      }
      frame "Adjust Plot scales etc" {
        n152 = Greater Than 0?(x=w387) -> (x > 0?=w386:bool)
        n153 = Array Size(array=w389) -> (size(s)=w405:i32)
        n154 = property on="XY Graph" class="XYGraph (strict)"("Legend:Plots Shown"=w405) -> ()  [unwired: 2 in, 2 out]
        n155 = Build Array(u8 6 ("Write Attribute"), u8 1 ("Write Attribute"), u8 11 ("Write Attribute"), u8 2 ("Write Attribute"), u8 5 ("Write Attribute"), u8 13 ("Write Attribute"), u8 15 ("Write Attribute"), u8 10 ("Write Attribute"), u8 12 ("Write Attribute"), u8 14 ("Write Attribute")) -> (w393:u8[])
        n156 = local read "No of Series"() -> (w388:i32)
        n157 = case shown="\"None\", Default" w384 {
          tunnel: ["Adjust plot scales2" "Show percentage change" ("t") "Set spectra axis" ("t") "Set spectra axis" ("t")] -> w383
          frame "None", Default {
          }
          frame "% change" {
          }
          frame "Spectrum" {
          }
          frame "Norm Spec" {
          }
        }
        n158 = Select(t=u8 2 ("Plot.Plot Interpolation"), s=w386, f=u8 0 ("Plot.Plot Interpolation")) -> (s? t:f=w390:u8)
        n159 = for {
          N: w388 -> [_]
          tunnel: w389 -> [w419] mode=indexing
          tunnel: w393 -> [w423]
          tunnel: w390 -> [w412]
          i -> [w422]
          w424 = u32 0
          n160 = String Length(string=w419) -> (length=w415:i32)
          n161 = Subtract(x=w415, y=2) -> (x-y=w413:i32)
          n162 = String Subset(string=w419, offset (0)=0, length (rest)=w413) -> (substring=w418:string)
          n163 = Concatenate Strings(w418, "  " ("string")) -> (w416:string)
          n164 = Index Array(array=w423, index=w422) -> (element=w421:u8)
          n165 = property on="XY Graph" class="XYGraph (strict)"("Active Plot"=w422, "Plot.Plot Name"=w416, "Plot.Fill/Point Color"=w424, "Plot.Plot Color"=w424, "Plot.Point Style"=w421, "Plot.Line Style"=u8 0, "Plot.Plot Interpolation"=w412) -> ()  [unwired: 2 in, 2 out]
        }
        "XY Graph" <- w382
      }
      frame "Adjust plot scales2" {
        n166 = property on="XY Graph" class="XYGraph (strict)"("X Scale.Name Label.Text"=w426, "Y Scale.Name Label.Text"=w425, "Cursor.Visible"=FALSE) -> ()  [unwired: 2 in, 2 out]
      }
      frame "Show percentage change" {
        n167 = Concatenate Strings(w437, " % Change" ("string")) -> (w440:string)
        n168 = property on="XY Graph" class="XYGraph (strict)"("X Scale.Name Label.Text"=w438, "Y Scale.Name Label.Text"=w440, "Cursor.Visible"=FALSE) -> ()  [unwired: 2 in, 2 out]
      }
      frame "Set spectra axis" {
        n169 = case shown="\"Spectrum\", Default" w445 {
          tunnel: [" Spectral Energy" ("string") " Normalised Spectral Energy" ("string")] -> w453
          frame "Spectrum", Default {
          }
          frame "Norm Spec" {
          }
        }
        n170 = Concatenate Strings(w450, w453) -> (w452:string)
        n171 = property on="XY Graph" class="XYGraph (strict)"("X Scale.Name Label.Text"="Wavelength [mm]", "Y Scale.Name Label.Text"=w452, "Cursor.Visible"=FALSE) -> ()  [unwired: 2 in, 2 out]
      }
      frame "Fill Second legend" {
        n172 = global read "Results_plotter_Global.vi" "Current Data Filenames"() -> (w463:string)
        n173 = call "Fast_string_Replace.vi"("Replace match with:"="_", "Input String"=w463, "regular expression"="[/]") -> ("Output String"=w467:string)  [unwired: 2 out]
        n174 = call "Fast_string_Replace.vi"("Replace match with:"="_", "Input String"=w467, "regular expression"="__") -> ("Output String"=w464:string)  [unwired: 2 out]
        n175 = call "Fast_string_Replace.vi"("Replace match with:"="", "Input String"=w464, "regular expression"=" ") -> ("Output String"=w462:string)  [unwired: 2 out]
        n176 = String Subset(string=w462, offset (0)=0, length (rest)=30 ("length (rest)")) -> (substring=w461:string)
        n177 = Build Path(base path=w474, name or relative path=w461) -> (appended path=w478:path)
      }
      frame "Calculate plot max and min values" {
        n178 = local read "plot error bars?"() -> (w481:bool)
        n179 = for {
          tunnel: w509 -> [w537] mode=indexing
          shift-right: [w534] -> w505
          shift-left: _ -> [w530]
          shift-right: [w533] -> w506
          shift-left: _ -> [w529]
          shift-right: [w532] -> w500
          shift-left: _ -> [w528]
          shift-right: [w531] -> w499
          shift-left: _ -> [w527]
          tunnel: w482 -> [w525]
          tunnel: w481 -> [w526]
          tunnel: w480 -> [w523]
          i -> [w524]
          n180 = Unbundle(w537) -> ("Output"=w536:dbl[], w535:dbl[])
          n181 = case shown="False" w526 {
            tunnel: w525 -> [_ w558]
            tunnel: w524 -> [_ w557]
            tunnel: [0.0 w553] -> w518
            frame False {
            }
            frame True {
              n182 = Index Array(array=w558, index=w557) -> (element=w556:cluster{string[]})
              n183 = Unbundle(w556) -> (w555:string[])
              n184 = Fract/Exp String To Number(string=w555) -> (number=w554:dbl[])  [unwired: 4 out]
              n185 = Array Max & Min(array=w554) -> (max value=w553:dbl)  [unwired: 3 out]
            }
          }
          n186 = Array Max & Min(array=w536) -> (max value=w516:dbl, min value=w514:dbl)  [unwired: 2 out]
          n187 = Array Max & Min(array=w535) -> (max value=w522:dbl, min value=w520:dbl)  [unwired: 2 out]
          n188 = case shown="True" w523 {
            tunnel: w522 -> [w544 w551]
            tunnel: [w543 w551] -> w521
            tunnel: w520 -> [w542 w550]
            tunnel: [w541 w550] -> w519
            tunnel: w518 -> [w540 w549]
            tunnel: [w539 w545] -> w517
            tunnel: w516 -> [w539 w548]
            tunnel: [w538 w546] -> w515
            tunnel: w514 -> [w538 w547]
            frame False {
              n189 = Subtract(x=w542, y=w540) -> (x-y=w541:dbl)
              n190 = Add(x=w544, y=w540) -> (x+y=w543:dbl)
            }
            frame True {
              n191 = Add(x=w548, y=w549) -> (x+y=w545:dbl)
              n192 = Subtract(x=w547, y=w549) -> (x-y=w546:dbl)
            }
          }
          n193 = case shown="0" w524 {
            tunnel: [w562 w576] -> w534
            tunnel: w517 -> [w562 w575]
            tunnel: w515 -> [w561 w572]
            tunnel: [w561 w571] -> w533
            tunnel: [w560 w564] -> w532
            tunnel: w521 -> [w560 w567]
            tunnel: [w559 w563] -> w531
            tunnel: w519 -> [w559 w565]
            tunnel: w530 -> [_ w577]
            tunnel: w529 -> [_ w574]
            tunnel: w528 -> [_ w568]
            tunnel: w527 -> [_ w566]
            frame 0 {
            }
            frame 1, Default {
              n194 = Greater?(x=w568, y=w567) -> (0:w569:bool)
              n195 = Greater?(x=w577, y=w575) -> (0:w578:bool)
              n196 = Less?(x=w566, y=w565) -> (x < y?=w570:bool)
              n197 = Less?(x=w574, y=w572) -> (x < y?=w573:bool)
              n198 = Select(t=w568, s=w569, f=w567) -> (s? t:f=w564:dbl)
              n199 = Select(t=w566, s=w570, f=w565) -> (s? t:f=w563:dbl)
              n200 = Select(t=w577, s=w578, f=w575) -> (s? t:f=w576:dbl)
              n201 = Select(t=w574, s=w573, f=w572) -> (s? t:f=w571:dbl)
            }
          }
        }
        n202 = Subtract(x=w505, y=w506) -> (x-y=w507:dbl)
        n203 = Subtract(x=w500, y=w499) -> (x-y=w502:dbl)
        n204 = Multiply(x=w507, y=0.1) -> (x*y=w504:dbl)
        n205 = Multiply(x=w502, y=0.1) -> (x*y=w503:dbl)
        n206 = Add(x=w500, y=w503) -> (x+y=w485:dbl)
        n207 = Add(x=w505, y=w504) -> (x+y=w492:dbl)
        n208 = Subtract(x=w506, y=w504) -> (x-y=w489:dbl)
        n209 = Subtract(x=w499, y=w503) -> (x-y=w494:dbl)
        n210 = Select(t=w489, s="Xmin", f="Xmin Val") -> (s? t:f=w497:dbl)
        n211 = Select(t=w485, s="Ymax", f="Ymax Val") -> (s? t:f=w483:dbl)
        n212 = Select(t=w492, s="Xmax", f="Xmax Val") -> (s? t:f=w490:dbl)
        n213 = Select(t=w494, s="Ymin", f="Ymin Val") -> (s? t:f=w498:dbl)
        n214 = property on="XY Graph" class="XYGraph (strict)"("X Scale.Range:Maximum"=w490, "X Scale.Range:Minimum"=w497, "Y Scale.Range:Maximum"=w483, "Y Scale.Range:Minimum"=w498) -> ()  [unwired: 2 in, 2 out]
      }
      frame "Sort out plot title" {
        n215 = local read "Summarise"() -> (w594:u16)
        n216 = Index Array(array=w589, index (col)=0 ("disabled index (col)")) -> (element=w588:string[])  [unwired: 1 in]
        n217 = case shown="1, Default" "Plot Title" {
          tunnel: [w641 w647] -> w587
          tunnel: "Plot Title" -> [w641 w646]
          tunnel: w589 -> [_ w651]
          tunnel: "Plot Title" -> [_ w650]
          tunnel: w594 -> [_ w644]
          frame 0 {
          }
          frame 1, Default {
            n218 = Decrement(x=w650) -> (x-1=w649:u16)
            n219 = Add(x=w644, y=u16 2) -> (x+y=w643:u16)
            n220 = Index Array(array=w651, index (row)=w649, index (col)=w643) -> (element=w654:string)
            n221 = Empty String/Path?(string/path=w646) -> (empty?=w648:bool)
            n222 = call "Fast_string_Replace.vi"("Replace match with:"="~ ", "Input String"=w654, "regular expression"=":") -> ("Output String"=w653:string)  [unwired: 2 out]
            n223 = call <vilib>:"Trim Whitespace.vi"("string"=w653) -> ("trimmed string"=w652:string)  [unwired: 1 in]
            n224 = call "Fast_string_Replace.vi"("Replace match with:"="~", "Input String"=w652, "regular expression"="_") -> ("Output String"=w642:string)  [unwired: 2 out]
            n225 = case shown="False" w648 {
              tunnel: [w660 w663] -> w647
              tunnel: w642 -> [w662 w663]
              tunnel: w646 -> [w661 _]
              frame False {
                n226 = Concatenate Strings(w661, " " ("string"), w662) -> (w660:string)
              }
              frame True {
              }
            }
          }
        }
        n227 = case shown="False" "Show Labels?" {
          tunnel: w589 -> [w608 _]
          tunnel: w588 -> [w607 _]
          tunnel: w587 -> [w605 w640]
          tunnel: [w606 w640] -> w586
          frame False {
            n228 = local read "Added labels"() -> (w609:i32[])
            n229 = Concatenate Strings(w605, "         " ("string")) -> (w604:string)
            n230 = for {
              tunnel: w609 -> [w633] mode=indexing
              tunnel: w608 -> [w634]
              shift-right: [w624] -> w606
              shift-left: w604 -> [w625]
              tunnel: w607 -> [w622]
              n231 = Index Array(array=w634, index (col)=2 ("index (row)")) -> (element=w632:string[])  [unwired: 1 in]
              n232 = Index Array(array=w622, index=w633) -> (element=w628:string)
              n233 = Index Array(array=w632, index=w633) -> (element=w619:string)
              n234 = call "Fast_string_Replace.vi"("Replace match with:"=" ", "Input String"=w628, "regular expression"=":") -> ("Output String"=w627:string)  [unwired: 2 out]
              n235 = call <vilib>:"Trim Whitespace.vi"("string"=w627) -> ("trimmed string"=w626:string)  [unwired: 1 in]
              n236 = Match Pattern(string=w619, regular expression=";") -> (offset past match=w615:i32)  [unwired: 4 out]
              n237 = Match Pattern(string=w619, regular expression=" to ") -> (offset past match=w616:i32)  [unwired: 4 out]
              n238 = Format Into String(format string="%s=%s", w626, w619) -> (resulting string=w611:string)  [unwired: 2 in, 1 out]
              n239 = Less Than 0?(x=w615) -> (x < 0?=w617:bool)
              n240 = Less Than 0?(x=w616) -> (x < 0?=w618:bool)
              n241 = And(x=w617, y=w618) -> (x .and. y?=w614:bool)
              n242 = call "Fast_string_Replace.vi"("Replace match with:"="~", "Input String"=w611, "regular expression"="_") -> ("Output String"=w610:string)  [unwired: 2 out]
              n243 = case shown="True" w614 {
                tunnel: w625 -> [w635 w639]
                tunnel: [w635 w638] -> w624
                tunnel: w610 -> [_ w637]
                frame False {
                }
                frame True {
                  n244 = Concatenate Strings(w639, "    " ("string"), w637) -> (w638:string)
                }
              }
            }
          }
          frame True {
          }
        }
        "Final Title" <- w586
        n245 = Current VI's Path() -> (path=w584:path)
        n246 = call "Running_as_top_level.vi"("Vi path name"=w584) -> ("Top Level"=w582:bool)  [unwired: 1 out]
        n247 = case shown="True" w582 {
          tunnel: [w598 w601] -> w581
          tunnel: w580 -> [w598 _]
          tunnel: ["Get Filename" ("t") "Create plot directory"] -> w579
          frame False {
          }
          frame True {
            n248 = local read "Path"() -> (w600:path)
            n249 = Strip Path(path=w600) -> (name=w599:string)  [unwired: 1 out]
            n250 = Build Path(base path=w600, name or relative path=w599) -> (appended path=w601:path)
          }
        }
      }
      frame "Get Filename" {
        n251 = local read "Final Title"() -> (w667:string)
        n252 = case shown="\"% change\"" w669 {
          tunnel: ["" "Per_" "Spec_" "N_Spec_"] -> w668
          frame "None" {
          }
          frame "% change" {
          }
          frame "Spectrum" {
          }
          frame "Norm Spec" {
          }
        }
        n253 = Concatenate Strings(w668, w667) -> (w664:string)
        n254 = String Length(string=w667) -> (length=w666:i32)
        n255 = case shown="1, Default" w666 {
          tunnel: [w684 w685] -> w665
          tunnel: w664 -> [w684 w687]
          frame 0 {
          }
          frame 1, Default {
            n256 = Concatenate Strings(w687, "_") -> (w685:string)
          }
        }
        n257 = call "Auto_filename.vi"("Filename Max length"="Filename Max length", "Prefix"=w665) -> ("Filename"=w671:string)
        n258 = Build Path(base path=w678, name or relative path=w671) -> (appended path=w675:path)
        n259 = File/Directory Info(path=w675) -> (error out=w676:errorcluster)  [unwired: 1 in, 6 out]
        n260 = Build Path(base path=w675, name or relative path=w671) -> (appended path=w682:path)
        n261 = Unbundle By Name(w676) -> ("status"=w674:bool)
        n262 = Select(t="Create plot directory", s=w674, f="Find a unique name") -> (s? t:f=w681:string)
      }
      frame "Find a unique name" {
        n263 = Strip Path(path=w699) -> (stripped path=w698:path, name=w697:string)
        n264 = Strip Path(path=w698) -> (stripped path=w695:path)  [unwired: 1 out]
        n265 = List Folder(path=w695) -> (folder names=w696:string[])  [unwired: 1 in, 5 out]
        n266 = while {
          tunnel: w697 -> [w720]
          tunnel: 27 ("Max Length") -> [w719]
          tunnel: [w708] -> w694
          tunnel: w696 -> [w709]
          i -> [w710]
          stop <- w706 continue-if-true
          n267 = Add(x=97, y=w710) -> (x+y=w717:i32)
          n268 = Build Array(w717) -> (w718:i32[])
          n269 = Byte Array To String(unsigned byte array=w718) -> (string=w715:string)
          n270 = Concatenate Strings(w720, w715) -> (w713:string)
          n271 = Reverse String(1:w713) -> (0:w714:string)
          n272 = String Subset(string=w714, offset (0)=0, length (rest)=w719) -> (substring=w712:string)
          n273 = Reverse String(1:w712) -> (0:w708:string)
          n274 = Search 1D Array(1D array=w709, element=w708) -> (index of element=w707:i32)  [unwired: 1 out]
          n275 = Greater Or Equal To 0?(x=w707) -> (x >= 0?=w706:bool)
        }
        n276 = Build Path(base path=w695, name or relative path=w694) -> (appended path=w693:path)
        n277 = Build Path(base path=w693, name or relative path=w694) -> (appended path=w692:path)
      }
      frame "Create plot directory" {
        n278 = Strip Path(path=w723) -> (stripped path=→"Path":path)  [unwired: 1 out]
        n279 = case shown="True" "Save Automatically?" {
          tunnel: [w732 w734] -> w728
          tunnel: w723 -> [w732 w733]
          frame False {
          }
          frame True {
            n280 = call "Create_directory_path.vi"("Path name"=w733) -> ("Path name Out"=w734:path)  [unwired: 1 in, 1 out]
          }
        }
        n281 = Select(t="Save data analysis file", s="Save data analysis file", f="Save .dat file") -> (s? t:f=w726:string)
      }
      frame "Save data analysis file" {
        n282 = stacked-sequence {
          seq-local: [w746 _ _] -> [_ _ w790]
          seq-local: [_ w762 _] -> [_ _ w788]
          tunnel: w744 -> [_ _ w801]
          tunnel: [_ _ TRUE ("Top Level")] -> w743
          tunnel: [_ _ "Save .dat file"] -> w742
          tunnel: w741 -> [w749 w764 _]
          tunnel: w740 -> [_ _ _]
          tunnel: w739 -> [_ _ _]
          tunnel: w735 -> [_ w765 _]
          tunnel: w737 -> [w753 _ _]
          tunnel: w736 -> [w752 _ _]
          frame #0 {
            n283 = case shown="\"Norm Spec\"" w753 {
              tunnel: w752 -> [w756 w760]
              tunnel: [w755 w759] -> w751
              tunnel: ["Wavelength::[mm]" "Wavelength::[mm]"] -> w750
              frame "Spectrum", Default {
                n284 = Concatenate Strings(w756, ":Spectral:Energy") -> (w755:string)
              }
              frame "Norm Spec" {
                n285 = Concatenate Strings(w760, ":Normalised Spectral:Energy") -> (w759:string)
              }
            }
            n286 = Index Array(array=w749, index (col)=0 ("disabled index (col)")) -> (element=w747:string[])  [unwired: 1 in]
            n287 = Build Array (concatenate)(w750, w751, w747) -> (w746:string[])
          }
          frame #1 {
            n288 = for {
              tunnel: w765 -> [w776] mode=indexing
              tunnel: w764 -> [w773]
              shift-right: [w767] -> w762
              shift-left: string[][] [] -> [w766]
              i -> [w771]
              n289 = Unbundle(w776) -> ("Output"=w775:dbl[], w774:dbl[])
              n290 = Add(x=3 ("disabled index (col)"), y=w771) -> (x+y=w770:i32)
              n291 = Index Array(array=w773, index (col)=w770) -> (element=w769:string[])  [unwired: 1 in]
              n292 = for {
                tunnel: w775 -> [w782] mode=indexing
                tunnel: w774 -> [w781] mode=indexing
                tunnel: w769 -> [w778]
                tunnel: [w777] -> w768 mode=indexing
                n293 = call "Number_2_string.vi"("number"=w782) -> ("String"=w780:string)  [unwired: 1 in]
                n294 = call "Number_2_string.vi"("number"=w781) -> ("String"=w779:string)  [unwired: 1 in]
                n295 = Build Array (concatenate)(w780, w779, w778) -> (w777:string[])
              }
              n296 = Build Array (concatenate)(w766, w768) -> (w767:string[][])
            }
          }
          frame #2 {
            w797 = FALSE  # Append last row only
            w796 = FALSE  # exists?
            n297 = Strip Path(path=w801) -> (stripped path=w802:path, name=w804:string)
            n298 = Array Size(array=w788) -> (size(s)=w787:i32[])
            n299 = Concatenate Strings(w804, ".xls" ("string")) -> (w803:string)
            n300 = Index Array(array=w787, index=0) -> (element=w785:i32)
            n301 = Build Path(base path=w802, name or relative path=w803) -> (appended path=w791:path)
            n302 = Initialize Array("", w785) -> (w784:string[])
            n303 = Build Array (concatenate)(w784, w788) -> (w789:string[][])
            n304 = Initialize Array("", 10 ("Dimension Size")) -> (w795:string[])
            n305 = call "Asterisk_header.vi"("Channel names"=w795) -> ("Header string"=w792:string)
            n306 = call "Write_Ch_data_file.vi"("Append last row only"=w797, "Header string"=w792, "exists?"=w796, "Channel Values"=w789, "Channel names"=w790, "Filename"=w791) -> ()  [unwired: 2 in, 4 out]
          }
        }
      }
      frame "Save .dat file" {
        n307 = stacked-sequence {
          seq-local: [w819 _ _ _ _] -> [_ _ _ _ w939]
          seq-local: [_ w845 _ _ _] -> [_ _ _ _ w940]
          seq-local: [_ _ _ w878 _] -> [_ _ _ _ w941]
          seq-local: [_ _ w862 _ _] -> [_ _ _ w876 _]
          seq-local: [_ _ w854 _ _] -> [_ _ _ w873 _]
          seq-local: [_ _ w856 _ _] -> [_ _ _ w872 _]
          tunnel: w817 -> [_ _ _ _ w944]
          tunnel: [_ _ _ _ TRUE ("Top Level")] -> w816
          tunnel: [_ _ _ _ "Gnuplot script Start"] -> w815
          tunnel: w814 -> [w824 _ _ _ _]
          tunnel: w813 -> [_ w848 _ _ _]
          tunnel: w812 -> [_ w844 _ _ _]
          tunnel: w811 -> [_ _ _ w880 _]
          tunnel: w810 -> [_ _ _ w877 _]
          tunnel: w809 -> [_ w842 _ _ _]
          tunnel: [_ _ _ w875 _] -> w808
          tunnel: w807 -> [_ _ w860 _ _]
          tunnel: w806 -> [_ _ _ w874 _]
          tunnel: w805 -> [_ _ w857 _ _]
          frame #0 {
            n308 = Array Subset(array=w824, length (col)=3 ("length")) -> (w822:string[][])  [unwired: 3 in]
            n309 = Build Array("Column Name", "Numeric Tolerance", "Range of Values") -> (w828:string[])
            n310 = Build Array (concatenate)(w828, w822) -> (w820:string[][])
            n311 = for {
              shift-right: [w832] -> w819
              shift-left: "" -> [w829]
              tunnel: w820 -> [w833] mode=indexing
              n312 = for {
                shift-right: [w834] -> w831
                shift-left: w829 -> [w841]
                tunnel: w833 -> [w835] mode=indexing
                i -> [w840]
                n313 = Equal To 0?(x=w840) -> (x = 0?=w839:bool)
                n314 = Select(t="#", s=w839, f="\t") -> (s? t:f=w836:string)
                n315 = Concatenate Strings(w841, w836, w835) -> (w834:string)
              }
              n316 = Concatenate Strings(w831, "\n") -> (w832:string)
            }
          }
          frame #1 {
            w846 = "\n"
            n317 = case shown="\"% change\"" w842 {
              tunnel: w844 -> [w850 w852]
              tunnel: [w850 w851] -> w843
              frame "None", Default {
              }
              frame "% change" {
                n318 = Concatenate Strings(w852, " %" ("string")) -> (w851:string)
              }
            }
            n319 = Concatenate Strings(w846, w846, "#" ("string"), w848, "\t", w843, w846, w846) -> (w845:string)
          }
          frame #2 {
            n320 = global read "Results_plotter_Global.vi" "Precision"() -> (w859:string[])
            n321 = global read "Results_plotter_Global.vi" "Absisca"() -> (w858:i32)
            n322 = case shown="True" "Offset?" {
              tunnel: [0.0 w870] -> w863
              frame False {
              }
              frame True {
                n323 = property on="XY Graph" class="XYGraph (strict)"() -> ("Y Scale.Range:Maximum"=w869:dbl, "Y Scale.Range:Minimum"=w871:dbl)  [unwired: 2 in, 2 out]
                n324 = Subtract(x=w869, y=w871) -> (x-y=w870:dbl)
              }
            }
            "Profile offset" <- w863
            n325 = Index Array(array=w859, index=w858) -> (element=w855:string)
            n326 = case shown="False" w857 {
              tunnel: ["" w867] -> w856
              tunnel: w855 -> [w864 w867]
              tunnel: [w864 ""] -> w854
              frame False {
              }
              frame True {
              }
            }
            n327 = Multiply(x=w863, y=w860) -> (x*y=w862:dbl)
          }
          frame #3 {
            n328 = for {
              tunnel: w880 -> [w907] mode=indexing
              shift-right: [w906] -> w878
              shift-left: "" -> [w897]
              tunnel: w877 -> [w895] mode=indexing
              tunnel: w876 -> [w892]
              tunnel: [w898] -> w875 mode=indexing
              tunnel: w874 -> [w885] mode=indexing
              tunnel: w873 -> [w882]
              tunnel: w872 -> [w881]
              i -> [w902]
              w905 = "\n"
              n329 = Unbundle(w907) -> ("Output"=w900:dbl[], w901:dbl[])
              n330 = Multiply(x=w892, y=w902) -> (x*y=w887:dbl)
              n331 = Negate(x=w887) -> (-x=w886:dbl)
              n332 = call "Number_2_string.vi"("number"=w886) -> ("String"=w894:string)  [unwired: 1 in]
              n333 = Format Into String(format string="\\t%s\\tPlot offset", w894) -> (resulting string=w890:string)  [unwired: 2 in, 1 out]
              n334 = Equal To 0?(x=w887) -> (x = 0?=w891:bool)
              n335 = Select(t="", s=w891, f=w890) -> (s? t:f=w888:string)
              n336 = Unbundle(w885) -> (w884:string[])
              n337 = for {
                tunnel: w900 -> [w926] mode=indexing
                shift-right: [w914] -> w904
                shift-left: "" -> [w915]
                tunnel: w905 -> [w919]
                tunnel: w901 -> [w923] mode=indexing
                tunnel: w887 -> [w922]
                tunnel: [w921] -> w899 mode=indexing
                tunnel: w884 -> [w917]
                shift-right: [w913] -> _
                shift-left: string[] [] -> [w912]
                tunnel: w882 -> [w909]
                tunnel: w881 -> [w908]
                i -> [w918]
                w920 = "\t"
                n338 = Subtract(x=w923, y=w922) -> (x-y=w921:dbl)
                n339 = call "Number_2_string.vi"("precision"=w909, "number"=w926) -> ("String"=w925:string)
                n340 = call "Number_2_string.vi"("precision"=w908, "number"=w921) -> ("String"=w924:string)
                n341 = Index Array(array=w917, index=w918) -> (element=w916:string)
                n342 = Concatenate Strings(w925, w920, w924, w920, w916, w919) -> (w911:string)
                n343 = Search 1D Array(1D array=w912, element=w911) -> (index of element=w910:i32)  [unwired: 1 in]
                n344 = case shown="-1" w910 {
                  tunnel: w915 -> [w928 w933]
                  tunnel: [w928 w932] -> w914
                  tunnel: w911 -> [_ w929]
                  tunnel: w912 -> [w927 w931]
                  tunnel: [w927 w930] -> w913
                  frame 0, Default {
                  }
                  frame -1 {
                    n345 = Concatenate Strings(w933, w929) -> (w932:string)
                    n346 = Build Array (concatenate)(w931, w929) -> (w930:string[])
                  }
                }
              }
              n347 = Bundle("Output"=w900, w899) -> (w898:cluster{"Output":dbl[], dbl[]})  [unwired: 1 out]
              n348 = Concatenate Strings(w897, "#", w895, w888, w905, w904, w905, w905) -> (w906:string)
            }
          }
          frame #4 {
            w936 = FALSE  # advisory dialog? (display:T)
            w937 = FALSE  # append to file? (new file:F)
            n349 = Strip Path(path=w944) -> (stripped path=w945:path, name=w947:string)
            n350 = Concatenate Strings(w939, w940, w941) -> (w938:string)
            n351 = Concatenate Strings(w947, ".dat" ("string")) -> (w946:string)
            n352 = Build Path(base path=w945, name or relative path=w946) -> (appended path=w935:path)
            n353 = call "Write_Characters_To_File.vi"("file path (dialog if empty)"=w935, "advisory dialog? (display:T)"=w936, "character string"=w938, "append to file? (new file:F)"=w937) -> ()  [unwired: 1 in, 4 out]
          }
        }
      }
      frame "Gnuplot script Start" {
        n354 = case shown="\"% change\"" w976 {
          tunnel: w975 -> [w993 w996 w1000 w1004]
          tunnel: [w993 w995 w999 w1003] -> w972
          tunnel: [w992 w994 "Wavelength [mm]" ("X Axis Name") "Wavelength [mm]" ("X Axis Name")] -> w973
          tunnel: w974 -> [w992 w994 _ _]
          frame "None", Default {
          }
          frame "% change" {
            n355 = Concatenate Strings(w996, " % change" ("string")) -> (w995:string)
          }
          frame "Spectrum" {
            n356 = Concatenate Strings(w1000, " Spectral energy" ("string")) -> (w999:string)
          }
          frame "Norm Spec" {
            n357 = Concatenate Strings(w1004, " Normalised Spectral Energy" ("string")) -> (w1003:string)
          }
        }
        n358 = case shown="\"None\"" w953 {
          tunnel: [w983 w985 "Calculate fit parameters"] -> w952
          tunnel: "Edit Legend names" -> [w983 w985 _]
          tunnel: [w982 w984 w986] -> w950
          tunnel: "" -> [w982 w984 _]
          tunnel: "set parametric\n" -> [_ _ w986]
          frame "None" {
          }
          frame "Spline" {
          }
          frame "Linear", Default {
          }
        }
        n359 = local read "Final Title"() -> (w958:string)
        n360 = call "Text_for_latex.vi"("Input String"=w958) -> ("Output String"=w959:string)
        n361 = call "Text_for_latex.vi"("Input String"=w973) -> ("Output String"=w969:string)
        n362 = call "Text_for_latex.vi"("Input String"=w972) -> ("Output String"=w966:string)
        n363 = call "Fast_string_Replace.vi"("Replace match with:"="", "Input String"=w959, "regular expression"="[$]") -> ("Output String"=w957:string)  [unwired: 2 out]
        n364 = call "Fast_string_Replace.vi"("Replace match with:"="", "Input String"=w969, "regular expression"="[$]") -> ("Output String"=w965:string)  [unwired: 2 out]
        n365 = call "Fast_string_Replace.vi"("Replace match with:"="", "Input String"=w966, "regular expression"="[$]") -> ("Output String"=w964:string)  [unwired: 2 out]
        n366 = local read "Time format?"() -> (w954:bool)
        n367 = Format Into String(format string="set term epslatex color\nset output \"Plot.eps\"\n%sset xlabel '$%s$'\nset ylabel '$%s$'\nset samples 1000\nset title '$%s$' 0, 0\nset size %s,%s\n", w950, w965, w964, w957, "Graph width", "Graph Height") -> (resulting string=w956:string)  [unwired: 2 in, 1 out]
        n368 = case shown="True" w954 {
          tunnel: w956 -> [w988 w990]
          tunnel: [w988 w989] -> w955
          frame False {
          }
          frame True {
            n369 = Concatenate Strings(w990, "\nset xdata time\nset timefmt \"%s\"\nset format  x \"%d %H:%M\"\n") -> (w989:string)
          }
        }
      }
      frame "Calculate fit parameters" {
        # "k=1;    # label 1\nlab=\"23 mA\";\neval( sprintf (\"set label %d %s\", k, lab))"
        n370 = Strip Path(path=w1019) -> (name=w1018:string)  [unwired: 1 out]
        n371 = Select(t="2:1", s=w1007, f="1:2") -> (s? t:f=w1008:string)
        n372 = for {
          tunnel: w1021 -> [w1036]
          tunnel: w1018 -> [w1034]
          shift-right: [w1032] -> w1014
          shift-left: w1017 -> [w1033]
          tunnel: "Auto Zp" -> [w1031]
          tunnel: "Fixed Zp" -> [w1030]
          tunnel: w1008 -> [w1029]
          tunnel: w1007 -> [w1028]
          tunnel: w1006 -> [w1027] mode=indexing
          i -> [w1035]
          n373 = Unbundle(w1027) -> ("Output"=w1025:dbl[], w1023:dbl[])
          n374 = case shown="False" w1028 {
            tunnel: [w1038 w1040] -> w1026
            tunnel: w1025 -> [w1038 w1039]
            tunnel: [w1037 w1039] -> w1024
            tunnel: w1023 -> [w1037 w1040]
            frame False {
            }
            frame True {
            }
          }
          n375 = case shown="\"Gauss Lat\"" w1036 {
            tunnel: w1035 -> [w1049 w1069 w1085 w1104 w1128 w1132 w1138 w1144 _]
            tunnel: w1034 -> [w1051 w1070 w1079 w1109 w1129 w1133 w1139 w1145 _]
            tunnel: w1033 -> [w1059 w1074 w1094 w1119 w1127 w1135 w1141 w1147 w1149]
            tunnel: [w1058 w1073 w1093 w1118 w1126 w1134 w1140 w1146 w1149] -> w1032
            tunnel: w1031 -> [_ _ w1084 w1108 _ _ _ _ _]
            tunnel: w1030 -> [_ _ w1081 w1105 _ _ _ _ _]
            tunnel: w1029 -> [w1041 w1061 w1078 w1100 w1125 w1131 w1137 w1143 _]
            tunnel: w1026 -> [w1042 w1062 w1077 w1102 _ _ _ _ _]
            tunnel: w1024 -> [w1043 w1063 w1076 w1101 _ _ _ _ _]
            frame "Gauss Lat" {
              w1046 = 0.01  # A value of zero make gnuplot stop working
              n376 = Array Max & Min(array=w1043) -> (max value=w1053:dbl, max index (indices)=w1050:i32)  [unwired: 2 out]
              n377 = Array Max & Min(array=w1042) -> (max value=w1057:dbl, min value=w1056:dbl)  [unwired: 2 out]
              n378 = Index Array(array=w1042, index=w1050) -> (element=w1045:dbl)
              n379 = Subtract(x=w1057, y=w1056) -> (x-y=w1055:dbl)
              n380 = Divide(x=w1055, y=6.0) -> (x/y=w1052:dbl)
              n381 = Absolute Value(x=w1045) -> (abs(x)=w1047:dbl)
              n382 = Greater?(x=w1047, y=w1046) -> (0:w1048:bool)
              n383 = Select(t=w1045, s=w1048, f=w1046) -> (s? t:f=w1044:dbl)
              n384 = Format Into String(format string="\nf%d(t) = cmax%d*exp(-((t-offset%d)**2)/(2*sig%d**2))\ncmax%d = %.2f; sig%d = %.2f; offset%d = %.2f           # initial guess for cmax and sig and offset\nfit f%d(t) \"%s.dat\" index %d using %s via cmax%d, sig%d, offset%d #this is a gaussian fit\n", initial string=w1059, w1049, w1049, w1049, w1049, w1049, w1053, w1049, w1052, w1049, w1044, w1049, w1051, w1049, w1041, w1049, w1049, w1049) -> (resulting string=w1058:string)  [unwired: 1 in, 1 out]
            }
            frame "Guass glc" {
              w1066 = 0.01 ("y")
              n385 = Array Max & Min(array=w1063) -> (max value=w1072:dbl, max index (indices)=w1071:i32)  [unwired: 2 out]
              n386 = Index Array(array=w1062, index=w1071) -> (element=w1065:dbl)
              n387 = Absolute Value(x=w1065) -> (abs(x)=w1067:dbl)
              n388 = Greater?(x=w1067, y=w1066) -> (0:w1068:bool)
              n389 = Select(t=w1065, s=w1068, f=w1066) -> (s? t:f=w1064:dbl)
              n390 = Format Into String(format string="\nf%d(t) = cmax%d*((t/xmax%d)**(-(1+m%d)*q%d)*exp(((1+m%d)/2)*(1-(t/xmax%d)**(-2*q%d))))\ncmax%d = %.2f; xmax%d = %.2f; m%d = 1;  q%d = 0.73         # initial guess for cmax and xmax q and m\nfit f%d(t) \"%s.dat\" index %d using %s via cmax%d, xmax%d, m%d, q%d  #this is a gaussian fit\n", initial string=w1074, w1069, w1069, w1069, w1069, w1069, w1069, w1069, w1069, w1069, w1072, w1069, w1064, w1069, w1069, w1069, w1070, w1069, w1061, w1069, w1069, w1069, w1069) -> (resulting string=w1073:string)  [unwired: 1 in, 1 out]
            }
            frame "Gauss vert" {
              (unwired) "f1(x) = cmax1*exp(-((x-offset1)**2)/(2*sig1**2))"
              n391 = Array Max & Min(array=w1076) -> (max value=w1088:dbl, max index (indices)=w1086:i32)  [unwired: 2 out]
              n392 = Array Max & Min(array=w1077) -> (max value=w1092:dbl, min value=w1091:dbl)  [unwired: 2 out]
              n393 = Index Array(array=w1077, index=w1086) -> (element=w1083:dbl)
              n394 = Subtract(x=w1092, y=w1091) -> (x-y=w1090:dbl)
              n395 = Divide(x=w1090, y=6.0) -> (x/y=w1087:dbl)
              n396 = case shown="False" w1084 {
                tunnel: [w1097 w1099] -> w1082
                tunnel: w1083 -> [_ w1099]
                tunnel: w1081 -> [w1097 _]
                tunnel: [w1096 ""] -> w1080
                frame False {
                  w1096 = " #"  # #
                }
                frame True {
                }
              }
              n397 = Format Into String(format string="\nf%d(t) = cmax%d*(exp(-((t-Zp%d)**2)/(2*sigZ%d**2))+exp(-((t+Zp%d)**2)/(2*sigZ%d**2)))\ncmax%d = %.2f; sigZ%d = %.2f; Zp%d = %.2f           # initial guess for cmax and sig and offset\nfit f%d(t) \"%s.dat\" index %d using %s via cmax%d, sigZ%d%s, Zp%d #this is a gaussian fit\n", initial string=w1094, w1085, w1085, w1085, w1085, w1085, w1085, w1085, w1088, w1085, w1087, w1085, w1082, w1085, w1079, w1085, w1078, w1085, w1085, w1080, w1085) -> (resulting string=w1093:string)  [unwired: 1 in, 1 out]
            }
            frame "Gauss Vert with 2 sig" {
              n398 = Array Max & Min(array=w1101) -> (max value=w1111:dbl, max index (indices)=w1113:i32)  [unwired: 2 out]
              n399 = Array Max & Min(array=w1102) -> (max value=w1117:dbl, min value=w1116:dbl)  [unwired: 2 out]
              n400 = Index Array(array=w1102, index=w1113) -> (element=w1107:dbl)
              n401 = Subtract(x=w1117, y=w1116) -> (x-y=w1115:dbl)
              n402 = Divide(x=w1115, y=6.0) -> (x/y=w1110:dbl)
              n403 = call "Vert_Spread_2_Sig.vi"("Index"=w1104) -> ("resulting string"=w1112:string)
              n404 = case shown="True" w1108 {
                tunnel: [w1122 w1124] -> w1106
                tunnel: w1105 -> [w1122 _]
                tunnel: [w1121 ""] -> w1103
                tunnel: w1107 -> [_ w1124]
                frame False {
                  w1121 = " #"  # #
                }
                frame True {
                }
              }
              n405 = Format Into String(format string="\nf%d(t) = %s\ncmax%d = %.2f; sigZ_low%d = %.2f; sigZ_up%d = %.2f; Zp%d = %.2f           # initial guess for cmax and sig and offset\nfit f%d(t) \"%s.dat\" index %d using %s via cmax%d, sigZ_low%d, sigZ_up%d%s, Zp%d #this is a gaussian fit\n", initial string=w1119, w1104, w1112, w1104, w1111, w1104, w1110, w1104, w1110, w1104, w1106, w1104, w1109, w1104, w1100, w1104, w1104, w1104, w1103, w1104) -> (resulting string=w1118:string)  [unwired: 1 in, 1 out]
            }
            frame "2nd Ploy" {
              n406 = Format Into String(format string="\nf%d(t) = c%d*t**2 + b%d*t + a%d\n#a%d = 40; b%d = 300; c%d = 1           # initial guess for cmax and sig and offset\nfit f%d(t) \"%s.dat\" index %d using %s via a%d, b%d, c%d #this is a 2nd order poly fit\n", initial string=w1127, w1128, w1128, w1128, w1128, w1128, w1128, w1128, w1128, w1129, w1128, w1125, w1128, w1128, w1128) -> (resulting string=w1126:string)  [unwired: 1 in, 1 out]
            }
            frame "3rd Poly" {
              n407 = Format Into String(format string="\nf%d(t) = d%d*t**3 +c%d*t**2 + b%d*t + a%d\n#a%d = 40; b%d = 300; c%d = 1; d%d = 1         # initial guess for cmax and sig and offset\nfit f%d(t) \"%s.dat\" index %d using %s via a%d, b%d, c%d, d%d #this is a 3rd order poly fit\n", initial string=w1135, w1132, w1132, w1132, w1132, w1132, w1132, w1132, w1132, w1132, w1132, w1133, w1132, w1131, w1132, w1132, w1132, w1132) -> (resulting string=w1134:string)  [unwired: 1 in, 1 out]
            }
            frame "4th Poly" {
              n408 = Format Into String(format string="\nf%d(t) = e%d*t**4 + d%d*t**3 +c%d*t**2 + b%d*t + a%d\n#a%d = 40; b%d = 300; c%d = 1; d%d = 1  e%d = 1       # initial guess for cmax and sig and offset\nfit f%d(t) \"%s.dat\" index %d using %s via a%d, b%d, c%d, d%d, e%d #this is a 3rd order poly fit\n", initial string=w1141, w1138, w1138, w1138, w1138, w1138, w1138, w1138, w1138, w1138, w1138, w1138, w1138, w1139, w1138, w1137, w1138, w1138, w1138, w1138, w1138) -> (resulting string=w1140:string)  [unwired: 1 in, 1 out]
            }
            frame "Linear" {
              n409 = Format Into String(format string="\nf%d(t) = b%d*t + c%d\n#a%d = 40; b%d = 300; c%d = 1           # initial guess for cmax and sig and offset\nfit f%d(t) \"%s.dat\" index %d using %s via b%d, c%d #this is a Linear fit\n", initial string=w1147, w1144, w1144, w1144, w1144, w1144, w1144, w1144, w1145, w1144, w1143, w1144, w1144) -> (resulting string=w1146:string)  [unwired: 1 in, 1 out]
            }
            frame "Spline", Default {
            }
          }
        }
        n410 = Concatenate Strings(w1014, "save variables 'Coeff.txt'\n") -> (w1015:string)
      }
      frame "Edit Legend names" {
        n411 = local read "Profile offset"() -> (w1158:dbl)
        n412 = Multiply(x=w1160, y=w1158) -> (x*y=w1162:dbl)
        n413 = for {
          tunnel: w1168 -> [w1179] mode=indexing
          tunnel: [w1178] -> w1167 mode=indexing
          tunnel: [w1177] -> w1163
          i -> [w1177]
          n414 = String Length(string=w1179) -> (length=w1182:i32)
          n415 = Subtract(x=w1182, y=2) -> (x-y=w1180:i32)
          n416 = String Subset(string=w1179, length (rest)=w1180) -> (substring=w1170:string)  [unwired: 1 out]
          n417 = Match Pattern(string=w1170, regular expression="=") -> (before substring=w1174:string, after substring=w1171:string)  [unwired: 3 out]
          n418 = call "Match_Pat_Case_In.vi"("String to match"="legend", "String"=w1174) -> ("offset past match"=w1173:i32)  [unwired: 1 in, 3 out]
          n419 = Greater Than 0?(x=w1173) -> (x > 0?=w1172:bool)
          n420 = Select(t=w1171, s=w1172, f=w1170) -> (s? t:f=w1169:string)
          n421 = call "Text_for_latex.vi"("Input String"=w1169) -> ("Output String"=w1178:string)
        }
        n422 = Decrement(x=w1160) -> (x-1=w1159:dbl)
        n423 = Multiply(x=w1162, y=w1163) -> (x*y=w1157:dbl)
        n424 = Multiply(x=w1158, y=w1159) -> (x*y=w1156:dbl)
        n425 = Add(x=w1156, y=w1157) -> (x+y=→"Extra range":dbl)
        n426 = Equal To 0?(x="Legend Position") -> (x = 0?=w1153:bool)
        n427 = Select(t="Auto Legend Position", s=w1153, f="Specified Legend Position") -> (s? t:f=w1151:string)
      }
      frame "Auto Legend Position" {
        w1226 = "\n%sset key %s, %s spacing 1.0\n%s unset key\n"  # %sset key %s, %s spacing 1.0 %s unset key
        n428 = local read "Graph Height"() -> (w1201:string)
        n429 = property on="XY Graph" class="XYGraph (strict)"() -> ("X Scale.Range:Maximum"=w1186:dbl, "X Scale.Range:Minimum"=w1185:dbl, "Y Scale.Range:Minimum"=w1189:dbl, "Y Scale.Range:Maximum"=w1187:dbl)  [unwired: 2 in, 2 out]
        n430 = local read "Extra range"() -> (w1190:dbl)
        n431 = Fract/Exp String To Number(string=w1201) -> (number=w1200:dbl)  [unwired: 4 out]
        n432 = case shown="False" w1199 {
          tunnel: w1187 -> [w1236 w1240]
          tunnel: w1189 -> [w1235 w1239]
          tunnel: [w1236 w1238] -> w1219
          tunnel: [w1235 w1237] -> w1188
          frame False {
          }
          frame True {
            n433 = Logarithm Base 10(1:w1240) -> (0:w1238:dbl)
            n434 = Logarithm Base 10(1:w1239) -> (0:w1237:dbl)
          }
        }
        n435 = case shown="True" w1192 {
          tunnel: w1186 -> [w1230 w1234]
          tunnel: w1185 -> [w1229 w1233]
          tunnel: [w1230 w1232] -> w1207
          tunnel: [w1229 w1231] -> w1203
          frame False {
          }
          frame True {
            n436 = Logarithm Base 10(1:w1234) -> (0:w1232:dbl)
            n437 = Logarithm Base 10(1:w1233) -> (0:w1231:dbl)
          }
        }
        n438 = Divide(x=0.35 ("y"), y=w1200) -> (x/y=w1212:dbl)
        n439 = Subtract(x=w1188, y=w1190) -> (x-y=w1218:dbl)
        n440 = Subtract(x=w1207, y=w1203) -> (x-y=w1206:dbl)
        n441 = Subtract(x=w1219, y=w1218) -> (x-y=w1210:dbl)
        n442 = Divide(x=w1210, y=10.0) -> (x/y=w1208:dbl)
        "Delta y" <- w1208
        n443 = Multiply(x=-0.2, y=w1206) -> (x*y=w1204:dbl)
        n444 = Multiply(x=w1206, y=0.9) -> (x*y=w1222:dbl)
        n445 = Multiply(x=w1210, y=w1212) -> (x*y=w1221:dbl)
        n446 = Add(x=w1203, y=w1222) -> (x+y=w1194:dbl)
        n447 = Add(x=w1203, y=w1204) -> (x+y=→"X location":dbl)
        n448 = Subtract(x=w1218, y=w1221) -> (x-y=w1198:dbl)
        n449 = case shown="False" "Show legend?" {
          tunnel: "" -> [w1249 w1258]
          tunnel: "#" -> [w1248 w1257]
          tunnel: [w1248 w1258] -> w1214
          tunnel: [w1249 w1257] -> w1213
          tunnel: w1198 -> [w1247 w1255]
          tunnel: [w1247 w1253] -> w1183
          tunnel: w1208 -> [_ w1256]
          frame False {
          }
          frame True {
            n450 = local read "No of Series"() -> (w1252:i32)
            n451 = Add(x=0.65, y=w1252) -> (x+y=w1251:dbl)
            n452 = Multiply(x=w1256, y=w1251) -> (x*y=w1254:dbl)
            n453 = Subtract(x=w1255, y=w1254) -> (x-y=w1253:dbl)
          }
        }
        "Y location" <- w1183
        n454 = case shown="True" w1192 {
          tunnel: w1194 -> [w1241 w1243]
          tunnel: [w1241 w1242] -> w1193
          frame False {
          }
          frame True {
            n455 = Power Of 10(x=w1243) -> (10^x=w1242:dbl)
          }
        }
        n456 = case shown="True" w1199 {
          tunnel: w1198 -> [w1244 w1246]
          tunnel: [w1244 w1245] -> w1195
          frame False {
          }
          frame True {
            n457 = Power Of 10(x=w1246) -> (10^x=w1245:dbl)
          }
        }
        n458 = call "Number_2_string.vi"("number"=w1195) -> ("String"=w1196:string)  [unwired: 1 in]
        n459 = call "Number_2_string.vi"("number"=w1193) -> ("String"=w1197:string)  [unwired: 1 in]
        n460 = Format Into String(format string=w1226, initial string=w1224, w1214, w1197, w1196, w1213) -> (resulting string=w1225:string)  [unwired: 1 in, 1 out]
      }
      frame "Specified Legend Position" {
        w1289 = "\n%sset key %s  spacing 1.0\n%s unset key\n"  # %sset key %s  spacing 1.0 %s unset key
        n461 = local read "Graph Height"() -> (w1273:string)
        n462 = property on="XY Graph" class="XYGraph (strict)"() -> ("Y Scale.Range:Minimum"=w1267:dbl, "Y Scale.Range:Maximum"=w1265:dbl)  [unwired: 2 in, 2 out]
        n463 = local read "Extra range"() -> (w1268:dbl)
        n464 = Fract/Exp String To Number(string=w1273) -> (number=w1272:dbl)  [unwired: 4 out]
        n465 = case shown="True" w1271 {
          tunnel: w1265 -> [w1293 w1297]
          tunnel: w1267 -> [w1292 w1296]
          tunnel: [w1293 w1295] -> w1283
          tunnel: [w1292 w1294] -> w1266
          frame False {
          }
          frame True {
            n466 = Logarithm Base 10(1:w1297) -> (0:w1295:dbl)
            n467 = Logarithm Base 10(1:w1296) -> (0:w1294:dbl)
          }
        }
        n468 = local read "Show legend?"() -> (w1263:bool)
        n469 = local read "Legend Position"() -> (w1261:u16)
        n470 = property on="Legend Position" class="Ring (strict)"() -> ("Strings []"=w1260:string[])  [unwired: 2 in, 2 out]
        n471 = Divide(x=0.35 ("y"), y=w1272) -> (x/y=w1277:dbl)
        n472 = Subtract(x=w1266, y=w1268) -> (x-y=w1282:dbl)
        n473 = Index Array(array=w1260, index=w1261) -> (element=w1259:string)
        n474 = Subtract(x=w1283, y=w1282) -> (x-y=w1276:dbl)
        n475 = Divide(x=w1276, y=10.0) -> (x/y=w1274:dbl)
        n476 = Multiply(x=w1276, y=w1277) -> (x*y=w1285:dbl)
        n477 = Subtract(x=w1282, y=w1285) -> (x-y=w1270:dbl)
        n478 = case shown="True" w1263 {
          tunnel: "" -> [w1300 w1309]
          tunnel: "#" -> [w1299 w1308]
          tunnel: [w1299 w1309] -> w1279
          tunnel: [w1300 w1308] -> w1278
          tunnel: w1270 -> [w1298 w1306]
          tunnel: [w1298 w1304] -> w1262
          tunnel: w1274 -> [_ w1307]
          frame False {
          }
          frame True {
            n479 = local read "No of Series"() -> (w1303:i32)
            n480 = Add(x=0.65, y=w1303) -> (x+y=w1302:dbl)
            n481 = Multiply(x=w1307, y=w1302) -> (x*y=w1305:dbl)
            n482 = Subtract(x=w1306, y=w1305) -> (x-y=w1304:dbl)
          }
        }
        n483 = local write "Y location"(w1262) -> ()
        n484 = Format Into String(format string=w1289, initial string=w1287, w1279, w1259, w1278) -> (resulting string=w1288:string)  [unwired: 1 in, 1 out]
      }
      frame "Labels?" {
        n485 = local read "Show Labels?"() -> (w1320:bool)
        n486 = Array Size(array="Added labels") -> (size(s)=w1326:i32)
        n487 = Greater Than 0?(x=w1326) -> (x > 0?=w1322:bool)
        n488 = case shown="\"Y only\"" "Major Gridlines" {
          tunnel: ["" "xtics " "ytics " "xtics ytics "] -> w1311
          frame "None" {
          }
          frame "X only" {
          }
          frame "Y only" {
          }
          frame "Both X and Y" {
          }
        }
        n489 = case shown="\"Both X and Y\"" "Minor Gridlines" {
          tunnel: ["" "mxtics " "mytics " "mxtics mytics "] -> w1310
          frame "None" {
          }
          frame "X only" {
          }
          frame "Y only" {
          }
          frame "Both X and Y" {
          }
        }
        n490 = And(x=w1320, y=w1322) -> (x .and. y?=w1321:bool)
        n491 = Select(t="Add Labels to plot", s=w1321, f="Set plot ranges" ("t")) -> (s? t:f=w1323:string)
        n492 = Concatenate Strings(w1311, w1310) -> (w1314:string)
        n493 = Empty String/Path?(string/path=w1314) -> (empty?=w1313:bool)
        n494 = case shown="False" w1313 {
          tunnel: [w1334 ""] -> w1312
          tunnel: w1311 -> [w1333 _]
          tunnel: w1310 -> [w1332 _]
          frame False {
            n495 = Concatenate Strings("set grid ", w1333, w1332, "\n") -> (w1334:string)
          }
          frame True {
          }
        }
        n496 = Concatenate Strings(w1318, w1312) -> (w1317:string)
      }
      frame "Add Labels to plot" {
        n497 = stacked-sequence {
          seq-local: [w1355 _] -> [_ w1400]
          tunnel: [_ w1401] -> w1352
          tunnel: w1351 -> [_ w1402]
          tunnel: [_ "Set plot ranges" ("t")] -> w1348
          tunnel: w1347 -> [w1358 _]
          tunnel: w1346 -> [_ w1397]
          tunnel: w1345 -> [_ w1395]
          frame #0 {
            n498 = local read "Added labels"() -> (w1360:i32[])
            n499 = Index Array(array=w1358, index (col)=0 ("disabled index (col)")) -> (element=w1359:string[])  [unwired: 1 in]
            n500 = for {
              tunnel: w1360 -> [w1385] mode=indexing
              tunnel: w1359 -> [w1390]
              tunnel: w1358 -> [w1389]
              tunnel: "Summarise" -> [w1388]
              shift-right: [w1376] -> w1355
              shift-left: string[] [] -> [w1377]
              n501 = Add(x=w1388, y=u16 2) -> (x+y=w1386:u16)
              n502 = Index Array(array=w1389, index (col)=w1386) -> (element=w1384:string[])  [unwired: 1 in]
              n503 = Index Array(array=w1390, index=w1385) -> (element=w1381:string)
              n504 = Index Array(array=w1384, index=w1385) -> (element=w1375:string)
              n505 = call "Fast_string_Replace.vi"("Replace match with:"=" ", "Input String"=w1381, "regular expression"=":") -> ("Output String"=w1380:string)  [unwired: 2 out]
              n506 = call <vilib>:"Trim Whitespace.vi"("string"=w1380) -> ("trimmed string"=w1379:string)  [unwired: 1 in]
              n507 = Match Pattern(string=w1375, regular expression="=") -> (offset past match=w1373:i32)  [unwired: 4 out]
              n508 = Less Than 0?(x=w1373) -> (x < 0?=w1372:bool)
              n509 = Select(t="%s = %s" ("format string"), s=w1372, f="%s %s" ("format string")) -> (s? t:f=w1369:string)
              n510 = Format Into String(format string=w1369, w1379, w1375) -> (resulting string=w1362:string)  [unwired: 2 in, 1 out]
              n511 = Match Pattern(string=w1362, regular expression=";") -> (offset past match=w1367:i32)  [unwired: 4 out]
              n512 = Match Pattern(string=w1362, regular expression=" to ") -> (offset past match=w1366:i32)  [unwired: 4 out]
              n513 = Less Than 0?(x=w1367) -> (x < 0?=w1364:bool)
              n514 = Less Than 0?(x=w1366) -> (x < 0?=w1365:bool)
              n515 = And(x=w1364, y=w1365) -> (x .and. y?=w1363:bool)
              n516 = case shown="False" w1363 {
                tunnel: w1377 -> [w1391 w1394]
                tunnel: [w1391 w1392] -> w1376
                tunnel: w1362 -> [_ w1393]
                frame False {
                }
                frame True {
                  n517 = Build Array (concatenate)(w1394, w1393) -> (w1392:string[])
                }
              }
            }
          }
          frame #1 {
            n518 = local read "Show legend?"() -> (w1396:bool)
            n519 = local read "X location"() -> (w1399:dbl)
            n520 = local read "Delta y"() -> (w1398:dbl)
            n521 = for {
              shift-right: [w1423] -> w1401
              shift-left: w1402 -> [w1424]
              tunnel: w1400 -> [w1420] mode=indexing
              tunnel: w1399 -> [w1406]
              tunnel: w1398 -> [w1425]
              tunnel: w1397 -> [w1419]
              tunnel: w1396 -> [w1408]
              tunnel: w1395 -> [w1404]
              i -> [w1426]
              n522 = call "Text_for_latex.vi"("Input String"=w1420) -> ("Output String"=w1414:string)
              n523 = case shown="False" w1404 {
                tunnel: w1406 -> [w1429 w1431]
                tunnel: [w1429 w1430] -> w1405
                frame False {
                }
                frame True {
                  n524 = Power Of 10(x=w1431) -> (10^x=w1430:dbl)
                }
              }
              n525 = String Length(string=w1414) -> (length=w1417:i32)
              n526 = Less?(x=w1417, y=20) -> (x < y?=w1409:bool)
              n527 = Compound Arithmetic op=AND(w1409, invert w1408) -> (w1407:bool)
              n528 = Increment(x=w1426) -> (x+1=w1427:i32)
              n529 = case shown="True" w1407 {
                tunnel: [w1432 w1434] -> w1415
                tunnel: w1414 -> [w1432 w1435]
                tunnel: "~~~~~~~~~~~" -> [_ w1433]
                frame False {
                }
                frame True {
                  n530 = Concatenate Strings(w1433, w1435) -> (w1434:string)
                }
              }
              n531 = Multiply(x=w1426, y=w1425) -> (x*y=w1421:dbl)
              n532 = local read "Y location"() -> (w1422:dbl)
              n533 = call "Number_2_string.vi"("number"=w1405) -> ("String"=w1412:string)  [unwired: 1 in]
              n534 = Subtract(x=w1422, y=w1421) -> (x-y=w1418:dbl)
              n535 = case shown="False" w1419 {
                tunnel: w1418 -> [w1436 w1438]
                tunnel: [w1436 w1437] -> w1411
                frame False {
                }
                frame True {
                  n536 = Power Of 10(x=w1438) -> (10^x=w1437:dbl)
                }
              }
              n537 = call "Number_2_string.vi"("number"=w1411) -> ("String"=w1410:string)  [unwired: 1 in]
              n538 = Format Into String(format string="set label %d '%s' at %s, %s\n", initial string=w1424, w1427, w1415, w1412, w1410) -> (resulting string=w1423:string)  [unwired: 1 in, 1 out]
            }
          }
        }
      }
      frame "Set plot ranges" {
        (unwired) "set border"
        (unwired) "set nologscale  y"
        (unwired) "set logscale  y"
        w1474 = "#"
        w1475 = ""
        n539 = Select(t="\nset logscale  x\n", s=w1452, f=w1475) -> (s? t:f=w1449:string)
        n540 = property on="XY Graph" class="XYGraph (strict)"() -> ("X Scale.Range:Maximum"=w1471:dbl, "X Scale.Range:Minimum"=w1470:dbl, "Y Scale.Range:Maximum"=w1454:dbl, "Y Scale.Range:Minimum"=w1455:dbl)  [unwired: 2 in, 2 out]
        n541 = local read "Extra range"() -> (w1465:dbl)
        n542 = local read "Profile offset"() -> (w1461:dbl)
        n543 = Select(t="\nset logscale  y\n", s=w1457, f=w1475) -> (s? t:f=w1451:string)
        n544 = Decrement(x=w1460) -> (x-1=w1462:dbl)
        n545 = Multiply(x=w1461, y=w1462) -> (x*y=w1459:dbl)
        n546 = Add(x=w1459, y=w1454) -> (x+y=w1458:dbl)
        n547 = Subtract(x=w1455, y=w1465) -> (x-y=w1466:dbl)
        n548 = call "Number_2_string.vi"("number"=w1458) -> ("String"=w1443:string)  [unwired: 1 in]
        n549 = call "Number_2_string.vi"("number"=w1466) -> ("String"=w1444:string)  [unwired: 1 in]
        n550 = call "Number_2_string.vi"("number"=w1471) -> ("String"=w1445:string)  [unwired: 1 in]
        n551 = call "Gnuplot_offset_ytics.vi"("Separation"=w1460, "Mode"="Mode", "precision"="precision", "Legend"=w1463, "Max Plot Value"=w1454, "Profile offset"=w1461) -> ("concatenated string"=w1450:string)
        n552 = call "Number_2_string.vi"("number"=w1470) -> ("String"=w1446:string)  [unwired: 1 in]
        n553 = case shown="True" w1447 {
          tunnel: [w1485 w1487] -> w1441
          tunnel: w1446 -> [w1485 _]
          tunnel: [w1484 w1486] -> w1440
          tunnel: w1445 -> [w1484 _]
          tunnel: w1444 -> [_ w1487]
          tunnel: w1443 -> [_ w1486]
          frame False {
          }
          frame True {
          }
        }
        n554 = case shown="\"Linear\", Default" w1442 {
          tunnel: w1441 -> [_ w1482]
          tunnel: w1440 -> [_ w1481]
          tunnel: ["" w1480] -> w1439
          frame "Spline" {
          }
          frame "Linear", Default {
            n555 = Format Into String(format string="set trange [%s : %s]", w1482, w1481) -> (resulting string=w1480:string)  [unwired: 2 in, 1 out]
          }
        }
        n556 = Format Into String(format string="%s set xrange [%s : %s] \n%s set autoscale x \n%s set yrange [%s : %s]\n%s set autoscale y\n", initial string=w1473, w1475, w1446, w1445, w1474, w1475, w1444, w1443, w1474) -> (resulting string=w1468:string)  [unwired: 1 in, 1 out]
        n557 = Concatenate Strings(w1468, w1439, w1449, w1451, w1450) -> (w1469:string)
      }
      frame "Plot Command" {
        n558 = case shown="True" w1491 {
          tunnel: ["yerrorbars" "xerrorbars"] -> w1490
          tunnel: ["" ", t"] -> w1489
          tunnel: ["t, " ""] -> w1488
          frame False {
          }
          frame True {
          }
        }
        n559 = Strip Path(path=w1509) -> (name=w1510:string)  [unwired: 1 out]
        n560 = global read "Results_plotter_Global.vi" "Series Index"() -> (w1492:i32[])
        n561 = for {
          shift-right: [w1554] -> w1501
          shift-left: "\nplot " -> [w1555]
          tunnel: w1510 -> [w1556]
          tunnel: w1498 -> [w1553]
          tunnel: w1508 -> [w1548] mode=indexing
          tunnel: "Plot style" -> [w1549]
          tunnel: w1496 -> [w1536]
          tunnel: w1495 -> [w1547] mode=indexing
          tunnel: "plot error bars?" -> [w1543]
          tunnel: w1490 -> [w1526]
          tunnel: w1492 -> [w1521] mode=indexing
          tunnel: w1489 -> [w1519]
          tunnel: w1488 -> [w1518]
          i -> [w1520]
          n562 = Index Array(array=w1549, index=w1521) -> (element=w1530:u16)
          n563 = case shown="2" w1530 {
            tunnel: ["points" ("format string") "lines" ("format string") "linespoints" ("format string")] -> w1527
            frame 0, Default {
            }
            frame 1 {
            }
            frame 2 {
            }
          }
          n564 = Quotient & Remainder(x=w1521, y=8) -> (x-y*floor(x/y)=w1535:i32)  [unwired: 1 out]
          n565 = Index Array(array=w1536, index=w1535) -> (element=w1534:i32)
          n566 = case shown="\"Spline\"" w1553 {
            tunnel: w1520 -> [_ w1564 w1578 w1585 w1592 w1600 w1607 w1614 w1621 w1628]
            tunnel: w1556 -> [_ w1572 _ _ _ _ _ _ _ _]
            tunnel: ["" w1571 w1579 w1586 w1594 w1601 w1608 w1615 w1622 w1629] -> w1552
            tunnel: w1521 -> [_ w1563 w1577 w1583 w1591 w1599 w1606 w1613 w1620 w1627]
            tunnel: 2 -> [_ w1562 w1576 w1584 w1590 w1598 w1605 w1612 w1619 w1626]
            tunnel: w1519 -> [_ _ w1574 w1582 w1588 w1596 w1603 w1610 w1617 w1624]
            tunnel: w1518 -> [_ _ w1575 w1581 w1589 w1597 w1604 w1611 w1618 w1625]
            frame "None", Default {
            }
            frame "Spline" {
              n567 = Quotient & Remainder(x=w1564, y=2) -> (x-y*floor(x/y)=w1569:i32)  [unwired: 1 out]
              n568 = Equal To 0?(x=w1569) -> (x = 0?=w1568:bool)
              n569 = Select(t="1", s=w1568, f="2") -> (s? t:f=w1565:string)
              n570 = Format Into String(format string="\"%s.dat\" index %d using 1:2 axes x1y1 linecolor %d linetype %d title '' lt %s smooth csplines, ", w1572, w1564, w1563, w1562, w1565) -> (resulting string=w1571:string)  [unwired: 2 in, 1 out]
            }
            frame "Gauss Lat" {
              n571 = Format Into String(format string="%s cmax%d*exp(-((t-offset%d)**2)/(2*sig%d**2))%s  linecolor %d linetype %d title '', ", w1575, w1578, w1578, w1578, w1574, w1577, w1576) -> (resulting string=w1579:string)  [unwired: 2 in, 1 out]
            }
            frame "Gauss vert" {
              n572 = Format Into String(format string="%s cmax%d*(exp(-((t-Zp%d)**2)/(2*sigZ%d**2))+exp(-((t+Zp%d)**2)/(2*sigZ%d**2)))%s linecolor %d linetype %d title '', ", w1581, w1585, w1585, w1585, w1585, w1585, w1582, w1583, w1584) -> (resulting string=w1586:string)  [unwired: 2 in, 1 out]
            }
            frame "Gauss Vert with 2 sig" {
              n573 = call "Vert_Spread_2_Sig.vi"("Index"=w1592) -> ("resulting string"=w1593:string)
              n574 = Format Into String(format string="%s %s%s  linecolor %d linetype %d title '', ", w1589, w1593, w1588, w1591, w1590) -> (resulting string=w1594:string)  [unwired: 2 in, 1 out]
            }
            frame "Guass glc" {
              n575 = Format Into String(format string="%s cmax%d*((t/xmax%d)**(-(1+m%d)*q%d)*exp(((1+m%d)/2)*(1-(t/xmax%d)**(-2*q%d))))%s  linecolor %d linetype %d title '', ", w1597, w1600, w1600, w1600, w1600, w1600, w1600, w1600, w1596, w1599, w1598) -> (resulting string=w1601:string)  [unwired: 2 in, 1 out]
            }
            frame "2nd Ploy" {
              n576 = Format Into String(format string="%s c%d*t**2 + b%d*t + a%d%s  linecolor %d linetype %d title 'fit%d', ", w1604, w1607, w1607, w1607, w1603, w1606, w1605, w1607) -> (resulting string=w1608:string)  [unwired: 2 in, 1 out]
            }
            frame "3rd Poly" {
              n577 = Format Into String(format string="%s d%d*t**3  + c%d*t**2 + b%d*t + a%d %s linecolor %d linetype %d title 'fit%d', ", w1611, w1614, w1614, w1614, w1614, w1610, w1613, w1612, w1614) -> (resulting string=w1615:string)  [unwired: 2 in, 1 out]
            }
            frame "4th Poly" {
              n578 = Format Into String(format string="%s e%d*t**4 + d%d*t**3  + c%d*t**2 + b%d*t + a%d%s  linecolor %d linetype %d title 'fit%d', ", w1618, w1621, w1621, w1621, w1621, w1621, w1617, w1620, w1619, w1621) -> (resulting string=w1622:string)  [unwired: 2 in, 1 out]
            }
            frame "Linear" {
              n579 = Format Into String(format string="%s b%d*t + c%d%s  linecolor %d linetype %d title 'fit%d', ", w1625, w1628, w1628, w1624, w1627, w1626, w1628) -> (resulting string=w1629:string)  [unwired: 2 in, 1 out]
            }
          }
          n580 = call "Fast_string_Replace.vi"("Replace match with:"="", "Input String"=w1548, "regular expression"="[$]") -> ("Output String"=w1538:string)  [unwired: 2 out]
          n581 = Unbundle(w1547) -> (w1546:string[])
          n582 = Array Size(array=w1546) -> (size(s)=w1545:i32)
          n583 = Greater Than 0?(x=w1545) -> (x > 0?=w1544:bool)
          n584 = And(x=w1544, y=w1543) -> (x .and. y?=w1528:bool)
          n585 = Select(t=w1526, s=w1528, f=w1527) -> (s? t:f=w1525:string)
          n586 = Select(t=":3", s=w1528, f="") -> (s? t:f=w1539:string)
          n587 = Format Into String(format string="\"%s.dat\" index %d using 1:2%s axes x1y1 title '$%s$' with ", initial string=w1555, w1556, w1520, w1539, w1538) -> (resulting string=w1542:string)  [unwired: 1 in, 1 out]
          n588 = Format Into String(format string=" linecolor %d pointtype %d pointsize %.2f linetype %d, ", initial string=w1525, w1521, w1534, "Point Size", -1) -> (resulting string=w1529:string)  [unwired: 1 in, 1 out]
          n589 = Concatenate Strings(w1542, w1529, w1552, "\\" ("string"), "\n") -> (w1554:string)
        }
        n590 = String Length(string=w1501) -> (length=w1505:i32)
        n591 = Subtract(x=w1505, y=4) -> (x-y=w1503:i32)
        n592 = String Subset(string=w1501, length (rest)=w1503) -> (substring=w1502:string)  [unwired: 1 out]
        n593 = Concatenate Strings(w1507, w1502) -> (w1506:string)
      }
      frame "Write gnuplot file" {
        w1639 = FALSE  # append to file? (new file:F)
        w1640 = FALSE  # advisory dialog? (display:T)
        n594 = Strip Path(path=w1636) -> (stripped path=w1632:path)  [unwired: 1 out]
        n595 = Build Path(base path=w1632, name or relative path="gnuplot_script.txt") -> (appended path=w1641:path)
        n596 = call "gnuplot_legend.vi"("Plot style"=w1633, "Legend"=w1637) -> ()  [unwired: 1 out]
        n597 = call "Write_Characters_To_File.vi"("file path (dialog if empty)"=w1641, "advisory dialog? (display:T)"=w1640, "character string"=w1631, "append to file? (new file:F)"=w1639) -> ()  [unwired: 1 in, 4 out]
      }
      frame "Execute shell script" {
        n598 = call "Run_Gnuplot_Script.vi"("logfileName"=w1643, "workingDirectory"=w1644) -> ()
      }
      frame "Has pdf been generated?" {
        n599 = Strip Path(path=w1657) -> (stripped path=w1659:path, name=w1661:string)
        n600 = Concatenate Strings(w1661, ".pdf" ("string")) -> (w1660:string)
        n601 = Build Path(base path=w1659, name or relative path=w1660) -> (appended path=w1656:path)
        n602 = call "Does_file_exist_(simple).vi"("Pathname"=w1656) -> ("exists?"=w1655:bool)
        n603 = case shown="False" w1655 {
          tunnel: ["Open Standard output file" ("f") "Input Fit Coefficients into results file?"] -> w1650
          frame False {
          }
          frame True {
          }
        }
        n604 = Select(t="Show Re-Run Gnuplot?", s="Show Re-Run Gnuplot?", f=w1650) -> (s? t:f=w1651:string)
      }
      frame "Show Re-Run Gnuplot?" {
        n605 = Strip Path(path=w1668) -> (stripped path=w1667:path)  [unwired: 1 out]
        n606 = call "Re_run_Gnuplot.vi"("Plot folder (dialog if empty)"=w1667) -> ()  [unwired: 4 out]
      }
      frame "Input Fit Coefficients into results file?" {
        n607 = Greater?(x=w1678, y=T5."Spline") -> (0:w1676:bool)
        n608 = And(x="Put Coeff\nin Results file", y=w1676) -> (x .and. y?=w1674:bool)
      }
      frame "Read Fit Coefficients" {
        n609 = call "Fast_string_Replace.vi"("Replace match with:"="", "Input String"=w1691, "regular expression"=":") -> ("Output String"=w1688:string)  [unwired: 2 out]
        n610 = Strip Path(path=w1697) -> (stripped path=w1695:path)  [unwired: 1 out]
        n611 = Build Path(base path=w1695, name or relative path="Coeff.txt") -> (appended path=w1694:path)
        n612 = call "Read_File_Simple.vi"("Filename"=w1694) -> ("string"=w1692:string)  [unwired: 2 in, 7 out]
        n613 = for {
          tunnel: w1693 -> [w1715]
          tunnel: w1692 -> [w1712]
          tunnel: w1688 -> [w1711]
          tunnel: [w1709] -> w1687
          tunnel: w1686 -> [w1708] mode=indexing
          shift-right: [w1704] -> w1684
          shift-left: string[][] [] -> [w1705]
          i -> [w1714]
          n614 = case shown="\"Gauss vert\"" w1715 {
            tunnel: w1714 -> [_ w1736 w1740 w1756]
            tunnel: [string[] [] w1732 w1748 w1762] -> w1713
            tunnel: [string[] [] w1728 w1745 w1759] -> w1710
            frame "None", Default {
            }
            frame "Gauss Lat" {
              n615 = Format Into String(format string="sig%d", w1736) -> (resulting string=w1734:string)  [unwired: 2 in, 1 out]
              n616 = Format Into String(format string="offset%d", w1736) -> (resulting string=w1733:string)  [unwired: 2 in, 1 out]
              n617 = Format Into String(format string="cmax%d", w1736) -> (resulting string=w1735:string)  [unwired: 2 in, 1 out]
              n618 = Build Array(":Max:Lat", ":Sig Y:", ":Yo:") -> (w1728:string[])
              n619 = Build Array(w1735, w1734, w1733) -> (w1732:string[])
            }
            frame "Gauss Vert with 2 sig" {
              n620 = Format Into String(format string="Zp%d", w1740) -> (resulting string=w1749:string)  [unwired: 2 in, 1 out]
              n621 = Format Into String(format string="cmax%d", w1740) -> (resulting string=w1751:string)  [unwired: 2 in, 1 out]
              n622 = Format Into String(format string="sigZ_low%d", w1740) -> (resulting string=w1741:string)  [unwired: 2 in, 1 out]
              n623 = Format Into String(format string="sigZ_up%d", w1740) -> (resulting string=w1750:string)  [unwired: 2 in, 1 out]
              n624 = Build Array(":Max:Vert", ":Sig Z:Upper", ":Sig Z:Lower", ":Zp:") -> (w1745:string[])
              n625 = Build Array(w1751, w1750, w1741, w1749) -> (w1748:string[])
            }
            frame "Gauss vert" {
              n626 = Format Into String(format string="Zp%d", w1756) -> (resulting string=w1763:string)  [unwired: 2 in, 1 out]
              n627 = Format Into String(format string="cmax%d", w1756) -> (resulting string=w1764:string)  [unwired: 2 in, 1 out]
              n628 = Format Into String(format string="sigZ%d", w1756) -> (resulting string=w1755:string)  [unwired: 2 in, 1 out]
              n629 = Build Array(":Max:Vert", ":Sig Z:Upper", ":Sig Z:Lower", ":Zp:") -> (w1759:string[])
              n630 = Build Array(w1764, w1755, w1755, w1763) -> (w1762:string[])
            }
          }
          n631 = Unbundle(w1708) -> ("Output"=w1702:dbl[])  [unwired: 1 out]
          n632 = for {
            tunnel: w1713 -> [w1725] mode=indexing
            tunnel: w1712 -> [w1722]
            tunnel: [w1720] -> w1707 mode=indexing
            n633 = Concatenate Strings(w1725, " = " ("string")) -> (w1723:string)
            n634 = Match Pattern(string=w1722, regular expression=w1723) -> (after substring=w1721:string)  [unwired: 4 out]
            n635 = call "Split_at_return.vi"("String"=w1721) -> ("before substring"=w1720:string)  [unwired: 1 in, 3 out]
          }
          n636 = for {
            tunnel: w1711 -> [w1719]
            tunnel: w1710 -> [w1718] mode=indexing
            tunnel: [w1717] -> w1709 mode=indexing
            n637 = Concatenate Strings(w1719, w1718) -> (w1717:string)
          }
          n638 = Array Size(array=w1702) -> (size(s)=w1703:i32)
          n639 = for {
            N: w1703 -> [_]
            tunnel: w1707 -> [w1716]
            tunnel: [w1716] -> w1706 mode=indexing
          }
          n640 = Build Array (concatenate)(w1705, w1706) -> (w1704:string[][])
        }
        n641 = global write "Results_plotter_Global.vi" "New Chs In"(w1687) -> ()
        n642 = global write "Results_plotter_Global.vi" "New Values In"(w1684) -> ()
      }
      frame "Open Standard output file" {
        n643 = Strip Path(path=w1772) -> (stripped path=w1769:path)  [unwired: 1 out]
        n644 = Format Into String(format string="open \"%s\"", w1770) -> (resulting string=w1768:string)  [unwired: 2 in, 1 out]
        n645 = call <vilib>:"System Exec.vi"("working directory"=w1769, "command line"=w1768) -> ()  [unwired: 4 in, 6 out]
      }
    }
  }
  "Tex Info String" <- w17
  "Saved Automatically?" <- FALSE
